vi "Autonomous Independent.vi"() -> ()   [LabVIEW 2017]
doc: "This VI is called when autonomous begins, and will automatically be terminated when autonomous ends. You can carry out timed or sensor driven robot movement independently without needing to return to the caller."
uses:
  <vilib>/Rock Robotics/WPI/Solenoid/WPI_SolenoidValue.ctl
  <vilib>/Rock Robotics/WPI/Utilities/WPI_GetSetVariantRefNum.vi
  <vilib>/Rock Robotics/Network Tables/NT Read String.vi
  <vilib>/Rock Robotics/Network Tables/NT Write Numeric Array.vi
  <vilib>/Rock Robotics/WPI/Solenoid/WPI_SolenoidSetEnum.vi
  Desktop/2018 FINAL/E/2018 FINAL/C/Users/admin/Documents/LabVIEW Data/2018 FINAL CODE/Robot Global Data.vi
  <vilib>/addons/control/pid/pid.llb/PID (DBL).vi
  <vilib>/Rock Robotics/WPI/RobotDrive/WPI_RobotDriveArcadeDrive_Standard(NoSaturation).vi
  <vilib>/addons/control/pid/NI_PID_pid.lvlib
panel:
  out "Place 2 Scale":bool
  out "Place 1 Scale":bool
  out "Robots Decision 2":string
  out "Place Switch and Scale":bool
  out "Place 2 Switch":bool
  out "Center Place 1 Switch":bool
  out "Game Data":string
  out "Right":bool
  out "Center":bool
  out "Left":bool
  # "Be sure to right-click and choose Data Operations>>Make Current Value default if you want to save the array values with the VI"
types:
  T1 = enum16{"Drive Forward", "None", "Right", "Center", "Left"}
  T2 = typedef "WPI_JoystickDevRef.ctl" = cluster{"Device":T3}
  T3 = typedef "WPI_JoystickDeviceEnum.ctl" = enum16{"USB 0", "USB 1", "USB 2", "USB 3", "USB 4", "USB 5"}
  T4 = enum16{"Place 2 Scale Left", "Place 2 Scale Right", "Place Scale Right", "Place Switch and Scale Right", "Place 2 Switch Right", "Center Place 2 Switch Right", "Center Place 1 Switch Right", "Center Place 2 Switch Left", "Center Place 1 Switch Left", "Place Scale Left", "Place Switch and Scale Left", "Place 2 Switch Left", "Drive forward", "Do Nothing"}
  T5 = enum16{"Place 2 Scale", "Place 1 Scale", "Place Switch and Scale", "Place 2 Switch", "Center Place 2 Switch", "Center Place 1 Switch", "None"}
  T6 = typedef "WPI_SolenoidValue.ctl" = enum16{"Off", "On", "Forward", "Reverse"}
  T7 = cluster{"proportional gain (Kc)":dbl, "integral time (Ti, min)":dbl, "derivative time (Td, min)":dbl}
  T8 = typedef "WPI_RobotDriveDevRef.ctl" = cluster{"DevStatus":errorcluster, "Motors[]":T9[], "Square Inputs":bool, "Max Output":dbl}
  T9 = typedef "WPI_MotorControlDeviceRef.ctl" = cluster{"DeviceStatus":errorcluster, "Type":T10, "PWM":cluster{"PWM Channel":T11, "DeadBand":T12}, "CAN":cluster{"Device Number":u8, "SetOutput VI Ref":variant, "GetOutput VI Ref":variant, "Enable VI Ref":variant, "Disable VI Ref":variant, "Data":variant}, "Invert":bool, "DIO PWM":cluster{"PWM \"Enable\" Channel":T11, "DIOChannel":T13, "PWM Rate":dbl}}
  T10 = typedef "WPI_MotorControlType.ctl" = enum16{"PWM", "CAN", "DIO PWM"}
  T11 = typedef "FPGA_DIOPWMChannel.ctl" = enum8{"PWM 0", "PWM 1", "PWM 2", "PWM 3", "PWM 4", "PWM 5", "PWM 6", "PWM 7", "PWM 8", "PWM 9", "PWM MXP 0", "PWM MXP 1", "PWM MXP 2", "PWM MXP 3", "PWM MXP 4", "PWM MXP 5", "PWM MXP 6", "PWM MXP 7", "PWM MXP 8", "PWM MXP 9", "Invalid"}
  T12 = typedef "WPI_PWMDeadband.ctl" = cluster{"Name":string, "maxPositivePwm":i32, "minPositivePwm":i32, "centerPwm":i32, "maxNegativePwm":i32, "minNegativePwm":i32, "angularRange":u16}
  T13 = typedef "FPGA_DIOChannel.ctl" = enum8{"DIO 0", "DIO 1", "DIO 2", "DIO 3", "DIO 4", "DIO 5", "DIO 6", "DIO 7", "DIO 8", "DIO 9", "DIO MXP 0", "DIO MXP 1", "DIO MXP 2", "DIO MXP 3", "DIO MXP 4", "DIO MXP 5", "DIO MXP 6", "DIO MXP 7", "DIO MXP 8", "DIO MXP 9", "DIO MXP 10", "DIO MXP 11", "DIO MXP 12", "DIO MXP 13", "DIO MXP 14", "DIO MXP 15", "SPI Port CS1", "SPI Port CS2", "SPI Port CS3", "SPI Port MISO", "SPI Port MOSI", "Invalid"}
  T14 = typedef "CTRE_PigeonIMU_DeviceRef.ctl" = cluster{"DeviceStatus":errorcluster, "Device Number":u8, "Type":T15, "Device ID":u32, "Handle":u64, "UsageFrame":u32, "Library Path":path}
  T15 = typedef "CTRE_PigeonIMU_ConnectionType.ctl" = u32
  T16 = typedef "WPI_SolenoidDevRef.ctl" = cluster{"DevStatus":errorcluster, "Pneumatics Control Module":u8, "Forward Solenoid Channel":T17, "Reverse Solenoid Channel":T17}
  T17 = typedef "WPI_SolenoidChannel.ctl" = enum8{"Solenoid 0", "Solenoid 1", "Solenoid 2", "Solenoid 3", "Solenoid 4", "Solenoid 5", "Solenoid 6", "Solenoid 7", "Invalid"}
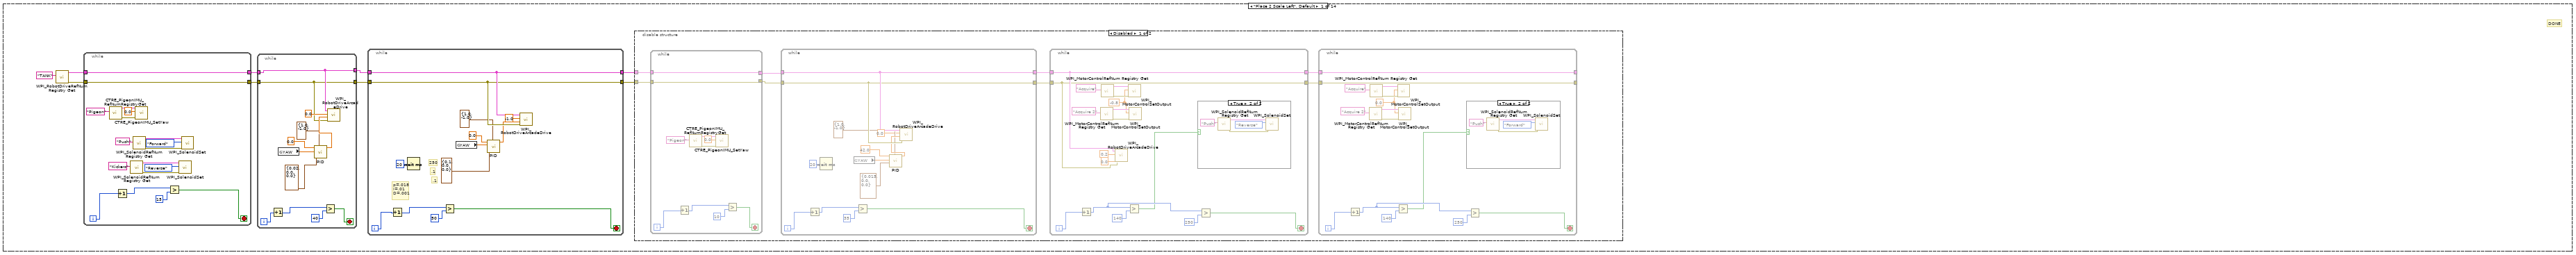
[diagram p2: hidden frame]
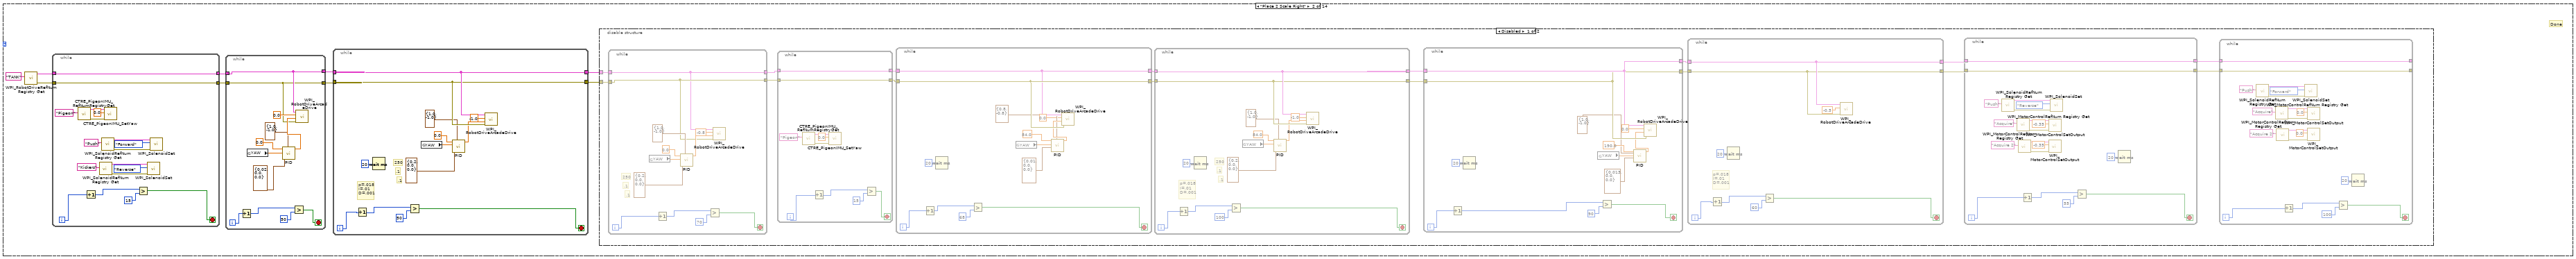
[diagram p6: hidden frame]
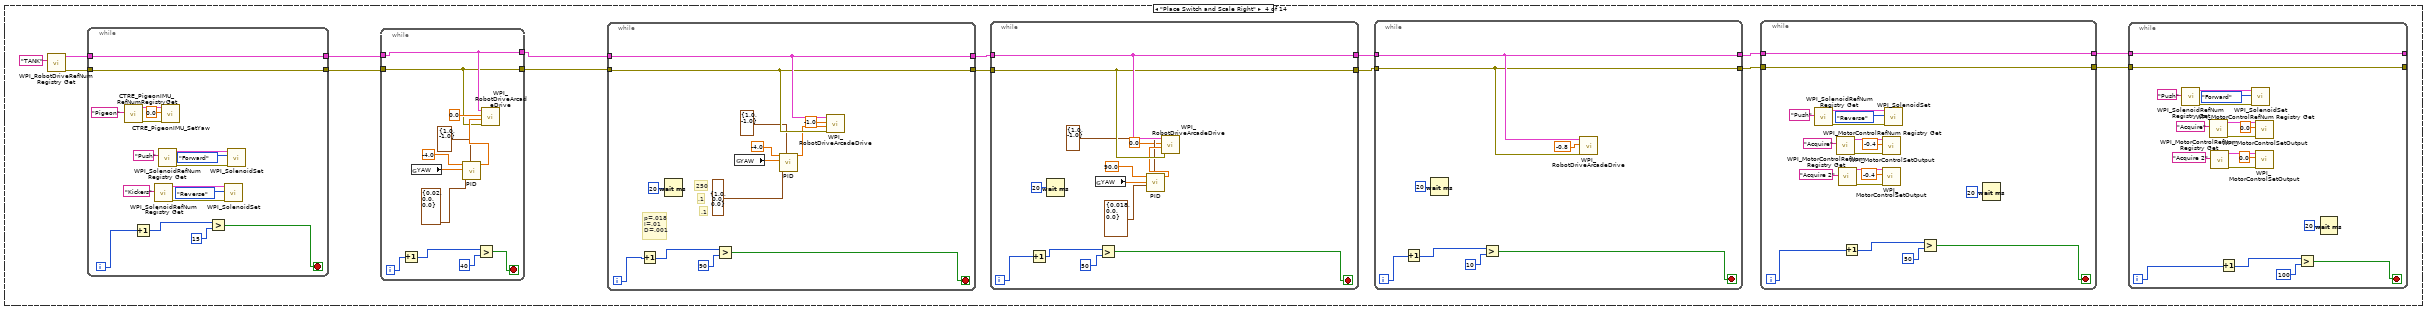
[diagram p10: hidden frame]
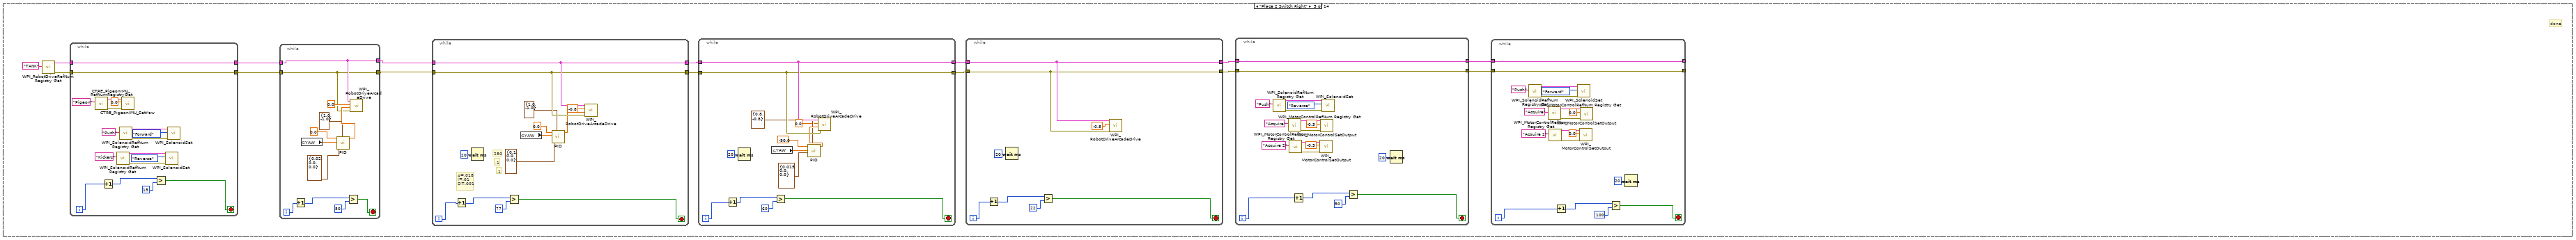
[diagram p11: hidden frame]
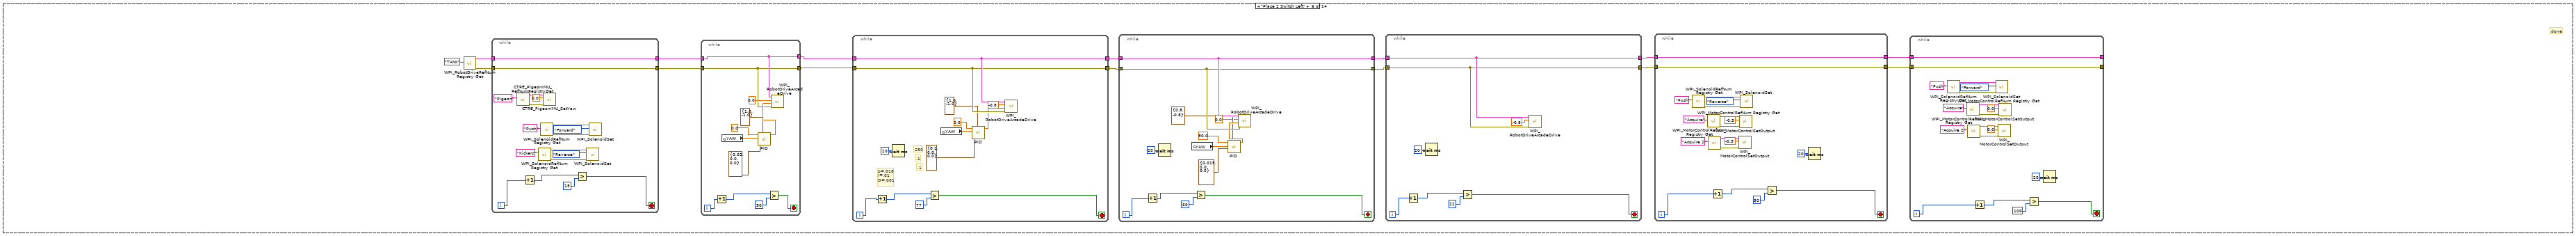
[diagram p12: hidden frame]
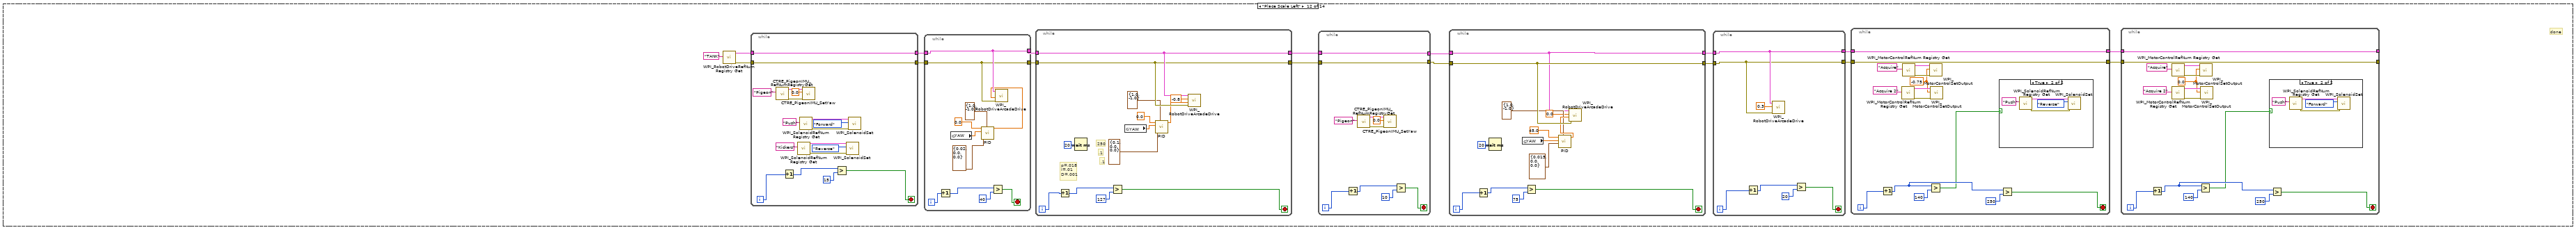
[diagram p18: hidden frame]
diagram:
  (unwired) "This function is run in parallel when the autonomous period begins. It will be terminated automatically when the period ends.\n\nNote that all Driver Station inputs are automatically latched and will not change once auto begins."
  # "5"
  # "LOGIC ALGORITHM"
  # "ALL AUTON STEPS GOES HERE"
  # "Players Choice"
  # "Order of difficulty"
  # "4"
  # "3"
  # "2"
  # "1"
  # "Game Data"
  # "Position"
  # "Position"
  # "LOGIC ALGORITHM"
  # "ALL AUTON STEPS GOES HERE"
  # "Position"
  # "This tells you the autonomous selected\nfrom the dashboard"
  # "Every 20ms, report that we are running autonomous\ncode. Loop will abort the same time as the VI."
  # "This gives you the joystick value\nthat is often the throttle"
  # "This tells you the driver position\nand alliance color"
  # "Possibilities"
  n1 = call <vilib>:"WPI_JoystickRefNum Registry Get.vi"("refnum name"="Auton") -> ("error out"=w43:errorcluster, "JoystickDevRef"=w44:T2)  [unwired: 9 in]
  n2 = call <vilib>:"WPI_JoystickGetValues.vi"("error in (no error)"=w43, "JoystickDevRef"=w44) -> ("Buttons"=w41:bool[])  [unwired: 5 in, 4 out]
  n3 = Index Array(array=w41) -> (element #1=w9:bool, element #2=w8:bool, element #4=w6:bool, element #5=w7:bool, element #10=w2:bool, element #11=w3:bool, element #13=w1:bool, element #14=w5:bool, element #16=w4:bool)  [unwired: 19 in, 10 out]
  "Left" <- w9
  "Center" <- w8
  "Right" <- w7
  "Center Place 1 Switch" <- w3
  "Place 2 Switch" <- w6
  "Place Switch and Scale" <- w2
  "Place 1 Scale" <- w5
  "Place 2 Scale" <- w4
  n4 = call <vilib>:"WPI_DriverStationGame Specific Data.vi"() -> ("Game Specific Data"=w10:string)  [unwired: 11 in]
  "Game Data" <- w10
  n5 = Select(t=T1."Right", s=w7, f=T1."None") -> (s? t:f=w37:T1)
  n6 = String Subset(string=w10, length (rest)=2 ("length (rest)")) -> (substring=w32:string)  [unwired: 1 in]
  n7 = Select(t=T1."Center", s=w8, f=w37) -> (s? t:f=w38:T1)
  n8 = Equal?(x=w32, y="RL") -> (x = y?=w26:bool)
  n9 = Equal?(x=w32, y="LR") -> (x = y?=w25:bool)
  n10 = Equal?(x=w32, y="LL") -> (x = y?=w28:bool)
  n11 = Equal?(x=w32, y="RR") -> (x = y?=w27:bool)
  n12 = Select(t=T1."Left", s=w9, f=w38) -> (s? t:f=w15:T1)
  n13 = Select(t=enum16{"None", "LR", "RL", "LL", "RR"}."LR", s=w25, f=enum16{"None", "LR", "RL", "LL", "RR"}."None") -> (s? t:f=w22:enum16{"None", "LR", "RL", "LL", "RR"})
  n14 = Select(t=enum16{"None", "LR", "RL", "LL", "RR"}."RL", s=w26, f=w22) -> (s? t:f=w23:enum16{"None", "LR", "RL", "LL", "RR"})
  n15 = Select(t=enum16{"None", "LR", "RL", "LL", "RR"}."RR", s=w27, f=w23) -> (s? t:f=w24:enum16{"None", "LR", "RL", "LL", "RR"})
  n16 = Select(t=enum16{"None", "LR", "RL", "LL", "RR"}."LL", s=w28, f=w24) -> (s? t:f=w16:enum16{"None", "LR", "RL", "LL", "RR"})
  n17 = Select(t=T1."Drive Forward", s=w1, f=w15) -> (s? t:f=w13:T1)
  n18 = case shown="\"Left\"" w13 {
    tunnel: w16 -> [_ _ w59 w163 w267]
    tunnel: w3 -> [_ _ w56 w159 w266]
    tunnel: w6 -> [_ _ w57 w160 w265]
    tunnel: w5 -> [_ _ w55 w161 w264]
    tunnel: w2 -> [_ _ w58 w162 w263]
    tunnel: w4 -> [_ _ w54 w157 w261]
    tunnel: [T4."Drive forward" T4."Do Nothing" w53 w158 w262] -> w11
    frame "Drive Forward", Default {
      # "Drive Forward code goes here. This is because drive forward can be done in any position on the field"
    }
    frame "None" {
      # "Nothing goes here."
    }
    frame "Right" {
      # "Game Data"
      n19 = case shown="\"LR\"" w59 {
        tunnel: w58 -> [w68 w88 w114 w134 _]
        tunnel: w55 -> [w73 w86 w112 w136 _]
        tunnel: w57 -> [w72 w85 w111 w137 _]
        tunnel: w56 -> [w71 w84 w110 w138 _]
        tunnel: w54 -> [w67 w87 w113 w135 _]
        tunnel: [w61 w89 w109 w132 T4."Do Nothing"] -> w53
        frame "RR" {
          # "Can do any auton"
          # "Right RR"
          n20 = Select(t=T5."Place Switch and Scale", s=w68, f=T5."None") -> (s? t:f=w69:T5)
          n21 = Select(t=T5."Place 2 Scale", s=w67, f=w69) -> (s? t:f=w76:T5)
          n22 = Select(t=T5."Place 1 Scale", s=w73, f=w76) -> (s? t:f=w75:T5)
          n23 = Select(t=T5."Place 2 Switch", s=w72, f=w75) -> (s? t:f=w74:T5)
          n24 = Select(t=T5."Place 1 Scale", s=w71, f=w74) -> (s? t:f=w70:T5)
          n25 = case shown="\"Place 2 Switch\"" w70 {
            tunnel: [T4."Place 2 Scale Right" T4."Place Scale Right" T4."Place Switch and Scale Right" T4."Place 2 Switch Right" T4."Do Nothing" T4."Do Nothing" T4."Do Nothing"] -> w61
            frame "Place 2 Scale", Default {
            }
            frame "Place 1 Scale" {
              # "Right switch"
            }
            frame "Place Switch and Scale" {
              # "Right Switch"
            }
            frame "Place 2 Switch" {
              # "Right Scale"
            }
            frame "Center Place 2 Switch" {
              # "Right Side"
            }
            frame "Center Place 1 Switch" {
            }
            frame "None" {
            }
          }
        }
        frame "LL" {
          # "Can do any auton"
          # "You can not score a cube so drive forward code goes here"
          # "Right LL"
          n26 = Select(t=T5."Place 2 Scale", s=w88, f=T5."None") -> (s? t:f=w96:T5)
          n27 = Select(t=T5."Place 2 Scale", s=w87, f=w96) -> (s? t:f=w100:T5)
          n28 = Select(t=T5."Place 2 Scale", s=w86, f=w100) -> (s? t:f=w99:T5)
          n29 = Select(t=T5."Place 2 Scale", s=w85, f=w99) -> (s? t:f=w98:T5)
          n30 = Select(t=T5."Place 2 Scale", s=w84, f=w98) -> (s? t:f=w97:T5)
          n31 = case shown="\"Place 2 Scale\", Default" w97 {
            tunnel: [T4."Drive forward" T4."Place Scale Left" T4."Place Switch and Scale Left" T4."Place 2 Switch Left" T4."Center Place 2 Switch Right" T4."Center Place 1 Switch Right" T4."Do Nothing"] -> w89
            frame "Place 2 Scale", Default {
            }
            frame "Place 1 Scale" {
              # "Right switch"
            }
            frame "Place Switch and Scale" {
            }
            frame "Place 2 Switch" {
            }
            frame "Center Place 2 Switch" {
            }
            frame "Center Place 1 Switch" {
            }
            frame "None" {
            }
          }
        }
        frame "RL" {
          # "Can do any auton"
          # "Right RL"
          n32 = Select(t=T5."Place 2 Switch", s=w114, f=T5."None") -> (s? t:f=w120:T5)
          n33 = Select(t=T5."Place 2 Switch", s=w113, f=w120) -> (s? t:f=w124:T5)
          n34 = Select(t=T5."Place 2 Switch", s=w112, f=w124) -> (s? t:f=w123:T5)
          n35 = Select(t=T5."Place 2 Switch", s=w111, f=w123) -> (s? t:f=w122:T5)
          n36 = Select(t=T5."Place 2 Switch", s=w110, f=w122) -> (s? t:f=w121:T5)
          n37 = case shown="\"Place 2 Switch\"" w121 {
            tunnel: [T4."Place 2 Scale Right" T4."Place Scale Right" T4."Place Switch and Scale Right" T4."Place 2 Switch Right" T4."Do Nothing" T4."Do Nothing" T4."Do Nothing"] -> w109
            frame "Place 2 Scale", Default {
            }
            frame "Place 1 Scale" {
              # "Right switch"
            }
            frame "Place Switch and Scale" {
              # "Right Switch"
            }
            frame "Place 2 Switch" {
              # "Right Scale"
            }
            frame "Center Place 2 Switch" {
              # "Right Side"
            }
            frame "Center Place 1 Switch" {
            }
            frame "None" {
            }
          }
        }
        frame "LR" {
          # "Can do any auton"
          # "Right LR"
          n38 = Select(t=T5."Place 1 Scale", s=w134, f=T5."None") -> (s? t:f=w144:T5)
          n39 = Select(t=T5."Place 1 Scale", s=w135, f=w144) -> (s? t:f=w148:T5)
          n40 = Select(t=T5."Place 1 Scale", s=w136, f=w148) -> (s? t:f=w147:T5)
          n41 = Select(t=T5."Place 1 Scale", s=w137, f=w147) -> (s? t:f=w146:T5)
          n42 = Select(t=T5."Place 1 Scale", s=w138, f=w146) -> (s? t:f=w145:T5)
          n43 = case shown="\"Place 1 Scale\"" w145 {
            tunnel: [T4."Place 2 Scale Right" T4."Place Scale Right" T4."Place Switch and Scale Right" T4."Place 2 Switch Right" T4."Do Nothing" T4."Do Nothing" T4."Do Nothing"] -> w132
            frame "Place 2 Scale", Default {
            }
            frame "Place 1 Scale" {
              # "Right switch"
            }
            frame "Place Switch and Scale" {
              # "Right Switch"
            }
            frame "Place 2 Switch" {
              # "Right Scale"
            }
            frame "Center Place 2 Switch" {
              # "Right Side"
            }
            frame "Center Place 1 Switch" {
            }
            frame "None" {
            }
          }
        }
        frame "None" {
          # "Nothing goes here."
        }
      }
    }
    frame "Center" {
      # "Game Data"
      n44 = case shown="\"LR\"" w163 {
        tunnel: w162 -> [w169 w193 w214 w239 _]
        tunnel: w161 -> [w167 w191 w215 w240 _]
        tunnel: w160 -> [w166 w190 w216 w241 _]
        tunnel: w159 -> [w165 w189 w217 w242 _]
        tunnel: [w164 w188 w212 w237 T4."Do Nothing"] -> w158
        tunnel: w157 -> [w168 w192 w213 w236 _]
        frame "RR" {
          # "Can do any auton"
          # "Center RR"
          n45 = Select(t=T5."Place 2 Switch", s=w169, f=T5."None") -> (s? t:f=w176:T5)
          n46 = Select(t=T5."Place 2 Switch", s=w168, f=w176) -> (s? t:f=w180:T5)
          n47 = Select(t=T5."Place 2 Switch", s=w167, f=w180) -> (s? t:f=w179:T5)
          n48 = Select(t=T5."Place 2 Switch", s=w166, f=w179) -> (s? t:f=w178:T5)
          n49 = Select(t=T5."Center Place 1 Switch", s=w165, f=w178) -> (s? t:f=w177:T5)
          n50 = case shown="\"Place 2 Scale\", Default" w177 {
            tunnel: [T4."Place 2 Scale Right" T4."Place Scale Right" T4."Place Switch and Scale Right" T4."Center Place 2 Switch Right" T4."Center Place 2 Switch Right" T4."Center Place 1 Switch Right" T4."Do Nothing"] -> w164
            frame "Place 2 Scale", Default {
            }
            frame "Place 1 Scale" {
              # "Right switch"
            }
            frame "Place Switch and Scale" {
              # "Right Switch"
            }
            frame "Place 2 Switch" {
            }
            frame "Center Place 2 Switch" {
            }
            frame "Center Place 1 Switch" {
            }
            frame "None" {
            }
          }
        }
        frame "LL" {
          # "Can do any auton"
          # "Center LL"
          n51 = Select(t=T5."Place 2 Switch", s=w193, f=T5."None") -> (s? t:f=w200:T5)
          n52 = Select(t=T5."Place 2 Switch", s=w192, f=w200) -> (s? t:f=w204:T5)
          n53 = Select(t=T5."Place 2 Switch", s=w191, f=w204) -> (s? t:f=w203:T5)
          n54 = Select(t=T5."Place 2 Switch", s=w190, f=w203) -> (s? t:f=w202:T5)
          n55 = Select(t=T5."Center Place 1 Switch", s=w189, f=w202) -> (s? t:f=w201:T5)
          n56 = case shown="\"None\"" w201 {
            tunnel: [T4."Place 2 Scale Right" T4."Place Scale Right" T4."Place Switch and Scale Right" T4."Center Place 2 Switch Left" T4."Center Place 2 Switch Left" T4."Center Place 1 Switch Left" T4."Do Nothing"] -> w188
            frame "Place 2 Scale", Default {
            }
            frame "Place 1 Scale" {
              # "Right switch"
            }
            frame "Place Switch and Scale" {
              # "Right Switch"
            }
            frame "Place 2 Switch" {
            }
            frame "Center Place 2 Switch" {
            }
            frame "Center Place 1 Switch" {
            }
            frame "None" {
            }
          }
        }
        frame "RL" {
          # "Can do any auton"
          # "Center RL"
          n57 = Select(t=T5."Place 2 Switch", s=w214, f=T5."None") -> (s? t:f=w224:T5)
          n58 = Select(t=T5."Place 2 Switch", s=w213, f=w224) -> (s? t:f=w228:T5)
          n59 = Select(t=T5."Place 2 Switch", s=w215, f=w228) -> (s? t:f=w227:T5)
          n60 = Select(t=T5."Place 2 Switch", s=w216, f=w227) -> (s? t:f=w226:T5)
          n61 = Select(t=T5."Center Place 1 Switch", s=w217, f=w226) -> (s? t:f=w225:T5)
          n62 = case shown="\"Center Place 1 Switch\"" w225 {
            tunnel: [T4."Place 2 Scale Right" T4."Place Scale Right" T4."Place Switch and Scale Right" T4."Center Place 2 Switch Right" T4."Center Place 2 Switch Right" T4."Center Place 1 Switch Right" T4."Do Nothing"] -> w212
            frame "Place 2 Scale", Default {
            }
            frame "Place 1 Scale" {
              # "Right switch"
            }
            frame "Place Switch and Scale" {
              # "Right Switch"
            }
            frame "Place 2 Switch" {
            }
            frame "Center Place 2 Switch" {
            }
            frame "Center Place 1 Switch" {
            }
            frame "None" {
            }
          }
        }
        frame "LR" {
          # "Can do any auton"
          # "Center LR"
          n63 = Select(t=T5."Place 2 Switch", s=w239, f=T5."None") -> (s? t:f=w248:T5)
          n64 = Select(t=T5."Place 2 Switch", s=w236, f=w248) -> (s? t:f=w252:T5)
          n65 = Select(t=T5."Place 2 Switch", s=w240, f=w252) -> (s? t:f=w251:T5)
          n66 = Select(t=T5."Place 2 Switch", s=w241, f=w251) -> (s? t:f=w250:T5)
          n67 = Select(t=T5."Center Place 1 Switch", s=w242, f=w250) -> (s? t:f=w249:T5)
          n68 = case shown="\"Center Place 1 Switch\"" w249 {
            tunnel: [T4."Place 2 Scale Right" T4."Place Scale Right" T4."Place Switch and Scale Right" T4."Center Place 2 Switch Left" T4."Center Place 2 Switch Left" T4."Center Place 1 Switch Left" T4."Do Nothing"] -> w237
            frame "Place 2 Scale", Default {
            }
            frame "Place 1 Scale" {
              # "Right switch"
            }
            frame "Place Switch and Scale" {
              # "Right Switch"
            }
            frame "Place 2 Switch" {
            }
            frame "Center Place 2 Switch" {
            }
            frame "Center Place 1 Switch" {
            }
            frame "None" {
            }
          }
        }
        frame "None" {
          # "Nothing goes here."
        }
      }
    }
    frame "Left" {
      n69 = case shown="\"LR\"" w267 {
        tunnel: w266 -> [w269 w292 w316 w340 _]
        tunnel: w265 -> [w270 w293 w317 w341 _]
        tunnel: w264 -> [w271 w294 w318 w342 _]
        tunnel: w263 -> [w273 w296 w320 w344 _]
        tunnel: [w268 w297 w321 w345 T4."Do Nothing"] -> w262
        tunnel: w261 -> [w272 w295 w319 w343 _]
        frame "RR" {
          # "Can do any auton"
          # "place 2 scale= drive across switch"
          # "Game Data"
          # "You can not score a cube so drive forward code goes here"
          # "Left RR"
          n70 = Select(t=T5."Place 2 Scale", s=w273, f=T5."None") -> (s? t:f=w280:T5)
          n71 = Select(t=T5."Place 2 Scale", s=w272, f=w280) -> (s? t:f=w284:T5)
          n72 = Select(t=T5."Place 2 Scale", s=w271, f=w284) -> (s? t:f=w283:T5)
          n73 = Select(t=T5."Place 2 Scale", s=w270, f=w283) -> (s? t:f=w282:T5)
          n74 = Select(t=T5."Place 2 Scale", s=w269, f=w282) -> (s? t:f=w281:T5)
          n75 = case shown="\"Place 2 Scale\", Default" w281 {
            tunnel: [T4."Drive forward" T4."Place Scale Left" T4."Place Switch and Scale Left" T4."Place 2 Switch Left" T4."Center Place 2 Switch Right" T4."Center Place 1 Switch Right" T4."Place 2 Scale Right"] -> w268
            frame "Place 2 Scale", Default {
            }
            frame "Place 1 Scale" {
              # "Right switch"
            }
            frame "Place Switch and Scale" {
            }
            frame "Place 2 Switch" {
            }
            frame "Center Place 2 Switch" {
            }
            frame "Center Place 1 Switch" {
            }
            frame "None" {
            }
          }
        }
        frame "LL" {
          # "Can do any auton"
          # "Left LL"
          n76 = Select(t=T5."Place Switch and Scale", s=w296, f=T5."None") -> (s? t:f=w304:T5)
          n77 = Select(t=T5."Place 2 Scale", s=w295, f=w304) -> (s? t:f=w308:T5)
          n78 = Select(t=T5."Place 1 Scale", s=w294, f=w308) -> (s? t:f=w307:T5)
          n79 = Select(t=T5."Place 2 Switch", s=w293, f=w307) -> (s? t:f=w306:T5)
          n80 = Select(t=T5."Place Switch and Scale", s=w292, f=w306) -> (s? t:f=w305:T5)
          n81 = case shown="\"Place 2 Switch\"" w305 {
            tunnel: [T4."Place 2 Scale Left" T4."Place Scale Left" T4."Place Switch and Scale Left" T4."Place 2 Switch Left" T4."Center Place 2 Switch Right" T4."Center Place 1 Switch Right" T4."Do Nothing"] -> w297
            frame "Place 2 Scale", Default {
            }
            frame "Place 1 Scale" {
              # "Right switch"
            }
            frame "Place Switch and Scale" {
            }
            frame "Place 2 Switch" {
            }
            frame "Center Place 2 Switch" {
            }
            frame "Center Place 1 Switch" {
            }
            frame "None" {
            }
          }
        }
        frame "RL" {
          # "Can do any auton"
          # "Left RL"
          n82 = Select(t=T5."Place 1 Scale", s=w320, f=T5."None") -> (s? t:f=w328:T5)
          n83 = Select(t=T5."Place 1 Scale", s=w319, f=w328) -> (s? t:f=w332:T5)
          n84 = Select(t=T5."Place 1 Scale", s=w318, f=w332) -> (s? t:f=w331:T5)
          n85 = Select(t=T5."Place 1 Scale", s=w317, f=w331) -> (s? t:f=w330:T5)
          n86 = Select(t=T5."Place 1 Scale", s=w316, f=w330) -> (s? t:f=w329:T5)
          n87 = case shown="\"Place 1 Scale\"" w329 {
            tunnel: [T4."Place 2 Scale Left" T4."Place Scale Left" T4."Place Switch and Scale Right" T4."Place 2 Switch Left" T4."Center Place 2 Switch Right" T4."Center Place 1 Switch Right" T4."Do Nothing"] -> w321
            frame "Place 2 Scale", Default {
            }
            frame "Place 1 Scale" {
              # "Right switch"
            }
            frame "Place Switch and Scale" {
              # "Right Switch"
            }
            frame "Place 2 Switch" {
            }
            frame "Center Place 2 Switch" {
            }
            frame "Center Place 1 Switch" {
            }
            frame "None" {
            }
          }
        }
        frame "LR" {
          # "Can do any auton"
          # "Left LR"
          n88 = Select(t=T5."Place 2 Switch", s=w344, f=T5."None") -> (s? t:f=w352:T5)
          n89 = Select(t=T5."Place 2 Switch", s=w343, f=w352) -> (s? t:f=w356:T5)
          n90 = Select(t=T5."Place 2 Switch", s=w342, f=w356) -> (s? t:f=w355:T5)
          n91 = Select(t=T5."Place 2 Switch", s=w341, f=w355) -> (s? t:f=w354:T5)
          n92 = Select(t=T5."Place 2 Switch", s=w340, f=w354) -> (s? t:f=w353:T5)
          n93 = case shown="\"Place 2 Switch\"" w353 {
            tunnel: [T4."Place 2 Scale Right" T4."Place Scale Right" T4."Place Switch and Scale Right" T4."Place 2 Switch Left" T4."Center Place 2 Switch Right" T4."Center Place 1 Switch Right" T4."Do Nothing"] -> w345
            frame "Place 2 Scale", Default {
            }
            frame "Place 1 Scale" {
              # "Right switch"
            }
            frame "Place Switch and Scale" {
              # "Right Switch"
            }
            frame "Place 2 Switch" {
            }
            frame "Center Place 2 Switch" {
            }
            frame "Center Place 1 Switch" {
            }
            frame "None" {
            }
          }
        }
        frame "None" {
          # "Nothing goes here."
        }
      }
    }
  }
  n94 = case shown="\"Place Scale Right\"" w11 {
    frame "Place 2 Scale Left", Default {
      # "DONE"
      n95 = call <vilib>:"WPI_RobotDriveRefNum Registry Get.vi"("refnum name"="TANK") -> ("error out"=w371:errorcluster, "RobotDriveDevRef"=w372:T8)  [unwired: 9 in]
      n96 = while {
        tunnel: [w474] -> w368
        tunnel: w372 -> [w474]
        tunnel: w371 -> [w473]
        tunnel: [w473] -> w366
        i -> [w470]
        stop <- w469 stop-if-true
        n97 = call <vilib>:"CTRE_PigeonIMU_RefNumRegistryGet.vi"("refnum name"="Pigeon") -> ("error out"=w466:errorcluster, "PigeonIMUDevRef"=w467:T14)  [unwired: 9 in]
        n98 = Increment(x=w470) -> (x+1=w471:i32)
        n99 = call <vilib>:"WPI_SolenoidRefNum Registry Get.vi"("refnum name"="Kickers") -> ("error out"=w458:errorcluster, "SolenoidDevRef"=w459:T16)  [unwired: 9 in]
        n100 = call <vilib>:"WPI_SolenoidRefNum Registry Get.vi"("refnum name"="Push") -> ("error out"=w462:errorcluster, "SolenoidDevRef"=w463:T16)  [unwired: 9 in]
        n101 = call <vilib>:"CTRE_PigeonIMU_SetYaw.vi"("error in (no error)"=w466, "Value"=0.0, "PigeonIMUDevRef"=w467) -> ()  [unwired: 7 in, 2 out]
        n102 = Greater?(x=w471, y=15) -> (0:w469:bool)
        n103 = call-poly <vilib>:"WPI_SolenoidSet.vi"("error in (no error)"=w458, "Value"=WPI_SolenoidValue."Reverse", "SolenoidDevRef"=w459) -> ()  [unwired: 7 in, 2 out]
        n104 = call-poly <vilib>:"WPI_SolenoidSet.vi"("error in (no error)"=w462, "Value"=WPI_SolenoidValue."Forward", "SolenoidDevRef"=w463) -> ()  [unwired: 7 in, 2 out]
      }
      n105 = while {
        tunnel: w368 -> [w446]
        tunnel: [w446] -> w367
        tunnel: w366 -> [w445]
        tunnel: [w445] -> w365
        i -> [w448]
        stop <- w447 stop-if-true
        n106 = Increment(x=w448) -> (x+1=w449:i32)
        n107 = global read "Robot Global Data.vi" "YAW"() -> (w454:dbl)
        n108 = call-poly <vilib>:"PID.vi"("output range"=cluster{"output high":dbl, "output low":dbl} {"output high"=1.0, "output low"=-1.0}, "PID gains"=T7 {"proportional gain (Kc)"=0.02, "integral time (Ti, min)"=0.0, "derivative time (Td, min)"=0.0}, "process variable"=w454, "setpoint"=0.0) -> ("output"=w453:dbl)  [unwired: 6 in, 1 out]
        n109 = Greater?(x=w449, y=40) -> (0:w447:bool)
        n110 = call-poly <vilib>:"WPI_RobotDriveArcadeDrive.vi"("error in (no error)"=w445, "Y axis value"=w453, "X axis value"=0.0, "RobotDriveDevRef"=w446) -> ()  [unwired: 5 in, 3 out]
      }
      n111 = while {
        tunnel: w367 -> [w482]
        tunnel: w365 -> [w481]
        tunnel: [w482] -> w370
        tunnel: [w481] -> w369
        i -> [w484]
        stop <- w487 stop-if-true
        # ".1"
        # ".1"
        # "250"
        # "p=.018\nI=.01\nD=.001"
        n112 = Increment(x=w484) -> (x+1=w483:i32)
        n113 = Wait (ms)(milliseconds to wait=u32 20) -> ()  [unwired: 1 out]
        n114 = Greater?(x=w483, y=50) -> (0:w487:bool)
        n115 = global read "Robot Global Data.vi" "YAW"() -> (w478:dbl)
        n116 = call-poly <vilib>:"PID.vi"("output range"=cluster{"output high":dbl, "output low":dbl} {"output high"=1.0, "output low"=-1.0}, "PID gains"=T7 {"proportional gain (Kc)"=0.1, "integral time (Ti, min)"=0.0, "derivative time (Td, min)"=0.0}, "process variable"=w478, "setpoint"=0.0) -> ("output"=w476:dbl)  [unwired: 6 in, 1 out]
        n117 = call-poly <vilib>:"WPI_RobotDriveArcadeDrive.vi"("error in (no error)"=w481, "Y axis value"=w476, "X axis value"=-1.0, "RobotDriveDevRef"=w482) -> ()  [unwired: 5 in, 3 out]
      }
      n118 = disable-structure shown="Disabled" {
        disable-tunnel: w370 -> [w379 _]
        disable-tunnel: w369 -> [w378 _]
        frame Disabled {
          n119 = while {
            tunnel: w379 -> [w409]
            tunnel: w378 -> [w410]
            tunnel: [w410] -> w377
            tunnel: [w409] -> w376
            i -> [w402]
            stop <- w401 stop-if-true
            n120 = Increment(x=w402) -> (x+1=w404:i32)
            n121 = call <vilib>:"CTRE_PigeonIMU_RefNumRegistryGet.vi"("refnum name"="Pigeon") -> ("error out"=w406:errorcluster, "PigeonIMUDevRef"=w407:T14)  [unwired: 9 in]
            n122 = call <vilib>:"CTRE_PigeonIMU_SetYaw.vi"("error in (no error)"=w406, "Value"=0.0, "PigeonIMUDevRef"=w407) -> ()  [unwired: 7 in, 2 out]
            n123 = Greater?(x=w404, y=10) -> (0:w401:bool)
          }
          n124 = while {
            tunnel: w376 -> [w439]
            tunnel: w377 -> [w438]
            tunnel: [w439] -> w381
            tunnel: [w438] -> w380
            i -> [w444]
            stop <- w443 stop-if-true
            n125 = Increment(x=w444) -> (x+1=w441:i32)
            n126 = Wait (ms)(milliseconds to wait=u32 20) -> ()  [unwired: 1 out]
            n127 = global read "Robot Global Data.vi" "YAW"() -> (w435:dbl)
            n128 = Greater?(x=w441, y=35) -> (0:w443:bool)
            n129 = call-poly <vilib>:"PID.vi"("output range"=cluster{"output high":dbl, "output low":dbl} {"output high"=1.0, "output low"=-1.0}, "PID gains"=T7 {"proportional gain (Kc)"=0.015, "integral time (Ti, min)"=0.0, "derivative time (Td, min)"=0.0}, "process variable"=w435, "setpoint"=42.0) -> ("output"=w434:dbl)  [unwired: 6 in, 1 out]
            n130 = call-poly <vilib>:"WPI_RobotDriveArcadeDrive.vi"("error in (no error)"=w438, "Y axis value"=w434, "X axis value"=0.0, "RobotDriveDevRef"=w439) -> ()  [unwired: 5 in, 3 out]
          }
          n131 = while {
            tunnel: w381 -> [w412]
            tunnel: w380 -> [w411]
            tunnel: [w412] -> w375
            tunnel: [w411] -> w374
            i -> [w427]
            stop <- w416 stop-if-true
            w419 = -0.8
            n132 = Increment(x=w427) -> (x+1=w417:i32)
            n133 = call <vilib>:"WPI_MotorControlRefNum Registry Get.vi"("refnum name"="Acquire 2") -> ("error out"=w420:errorcluster, "MotorControlDevRef"=w421:T9)  [unwired: 9 in]
            n134 = call <vilib>:"WPI_MotorControlRefNum Registry Get.vi"("refnum name"="Acquire") -> ("error out"=w423:errorcluster, "MotorControlDevRef"=w424:T9)  [unwired: 9 in]
            n135 = call-poly <vilib>:"WPI_RobotDriveArcadeDrive.vi"("error in (no error)"=w411, "Y axis value"=0.0, "X axis value"=0.2, "RobotDriveDevRef"=w412) -> ()  [unwired: 5 in, 3 out]
            n136 = Greater?(x=w417, y=140) -> (0:w415:bool)
            n137 = call <vilib>:"WPI_MotorControlSetOutput.vi"("error in (no error)"=w423, "Output"=w419, "MotorControlDevRef"=w424) -> ()  [unwired: 6 in, 3 out]
            n138 = call <vilib>:"WPI_MotorControlSetOutput.vi"("error in (no error)"=w420, "Output"=w419, "MotorControlDevRef"=w421) -> ()  [unwired: 6 in, 3 out]
            n139 = case shown="True" w415 {
              frame False {
              }
              frame True {
                n140 = call <vilib>:"WPI_SolenoidRefNum Registry Get.vi"("refnum name"="Push") -> ("error out"=w429:errorcluster, "SolenoidDevRef"=w430:T16)  [unwired: 9 in]
                n141 = call-poly <vilib>:"WPI_SolenoidSet.vi"("error in (no error)"=w429, "Value"=WPI_SolenoidValue."Reverse", "SolenoidDevRef"=w430) -> ()  [unwired: 7 in, 2 out]
              }
            }
            n142 = Greater?(x=w417, y=250) -> (0:w416:bool)
          }
          n143 = while {
            tunnel: w375 -> [w383]
            tunnel: w374 -> [w382]
            tunnel: [w383] -> _
            tunnel: [w382] -> _
            i -> [w396]
            stop <- w385 stop-if-true
            w388 = 0.0
            n144 = Increment(x=w396) -> (x+1=w386:i32)
            n145 = call <vilib>:"WPI_MotorControlRefNum Registry Get.vi"("refnum name"="Acquire 2") -> ("error out"=w389:errorcluster, "MotorControlDevRef"=w390:T9)  [unwired: 9 in]
            n146 = call <vilib>:"WPI_MotorControlRefNum Registry Get.vi"("refnum name"="Acquire") -> ("error out"=w392:errorcluster, "MotorControlDevRef"=w393:T9)  [unwired: 9 in]
            n147 = Greater?(x=w386, y=140) -> (0:w384:bool)
            n148 = call <vilib>:"WPI_MotorControlSetOutput.vi"("error in (no error)"=w392, "Output"=w388, "MotorControlDevRef"=w393) -> ()  [unwired: 6 in, 3 out]
            n149 = call <vilib>:"WPI_MotorControlSetOutput.vi"("error in (no error)"=w389, "Output"=w388, "MotorControlDevRef"=w390) -> ()  [unwired: 6 in, 3 out]
            n150 = case shown="True" w384 {
              frame False {
              }
              frame True {
                n151 = call <vilib>:"WPI_SolenoidRefNum Registry Get.vi"("refnum name"="Push") -> ("error out"=w398:errorcluster, "SolenoidDevRef"=w399:T16)  [unwired: 9 in]
                n152 = call-poly <vilib>:"WPI_SolenoidSet.vi"("error in (no error)"=w398, "Value"=WPI_SolenoidValue."Forward", "SolenoidDevRef"=w399) -> ()  [unwired: 7 in, 2 out]
              }
            }
            n153 = Greater?(x=w386, y=250) -> (0:w385:bool)
          }
        }
        frame Enabled {
        }
      }
    }
    frame "Place 2 Scale Right" {
      # "Done"
      n154 = call <vilib>:"WPI_RobotDriveRefNum Registry Get.vi"("refnum name"="TANK") -> ("error out"=w494:errorcluster, "RobotDriveDevRef"=w495:T8)  [unwired: 9 in]
      n155 = while {
        tunnel: [w649] -> w493
        tunnel: w495 -> [w649]
        tunnel: w494 -> [w648]
        tunnel: [w648] -> w492
        i -> [w645]
        stop <- w644 stop-if-true
        n156 = call <vilib>:"CTRE_PigeonIMU_RefNumRegistryGet.vi"("refnum name"="Pigeon") -> ("error out"=w641:errorcluster, "PigeonIMUDevRef"=w642:T14)  [unwired: 9 in]
        n157 = Increment(x=w645) -> (x+1=w646:i32)
        n158 = call <vilib>:"WPI_SolenoidRefNum Registry Get.vi"("refnum name"="Kickers") -> ("error out"=w633:errorcluster, "SolenoidDevRef"=w634:T16)  [unwired: 9 in]
        n159 = call <vilib>:"WPI_SolenoidRefNum Registry Get.vi"("refnum name"="Push") -> ("error out"=w637:errorcluster, "SolenoidDevRef"=w638:T16)  [unwired: 9 in]
        n160 = call <vilib>:"CTRE_PigeonIMU_SetYaw.vi"("error in (no error)"=w641, "Value"=0.0, "PigeonIMUDevRef"=w642) -> ()  [unwired: 7 in, 2 out]
        n161 = Greater?(x=w646, y=15) -> (0:w644:bool)
        n162 = call-poly <vilib>:"WPI_SolenoidSet.vi"("error in (no error)"=w633, "Value"=WPI_SolenoidValue."Reverse", "SolenoidDevRef"=w634) -> ()  [unwired: 7 in, 2 out]
        n163 = call-poly <vilib>:"WPI_SolenoidSet.vi"("error in (no error)"=w637, "Value"=WPI_SolenoidValue."Forward", "SolenoidDevRef"=w638) -> ()  [unwired: 7 in, 2 out]
      }
      n164 = while {
        tunnel: w493 -> [w621]
        tunnel: [w621] -> w491
        tunnel: w492 -> [w620]
        tunnel: [w620] -> w490
        i -> [w623]
        stop <- w622 stop-if-true
        n165 = Increment(x=w623) -> (x+1=w624:i32)
        n166 = global read "Robot Global Data.vi" "YAW"() -> (w629:dbl)
        n167 = call-poly <vilib>:"PID.vi"("output range"=cluster{"output high":dbl, "output low":dbl} {"output high"=1.0, "output low"=-1.0}, "PID gains"=T7 {"proportional gain (Kc)"=0.02, "integral time (Ti, min)"=0.0, "derivative time (Td, min)"=0.0}, "process variable"=w629, "setpoint"=0.0) -> ("output"=w628:dbl)  [unwired: 6 in, 1 out]
        n168 = Greater?(x=w624, y=50) -> (0:w622:bool)
        n169 = call-poly <vilib>:"WPI_RobotDriveArcadeDrive.vi"("error in (no error)"=w620, "Y axis value"=w628, "X axis value"=0.0, "RobotDriveDevRef"=w621) -> ()  [unwired: 5 in, 3 out]
      }
      n170 = while {
        tunnel: w491 -> [w657]
        tunnel: w490 -> [w656]
        tunnel: [w657] -> w489
        tunnel: [w656] -> w488
        i -> [w659]
        stop <- w662 stop-if-true
        # ".1"
        # ".1"
        # "250"
        # "p=.018\nI=.01\nD=.001"
        n171 = Increment(x=w659) -> (x+1=w658:i32)
        n172 = Wait (ms)(milliseconds to wait=u32 20) -> ()  [unwired: 1 out]
        n173 = Greater?(x=w658, y=50) -> (0:w662:bool)
        n174 = global read "Robot Global Data.vi" "YAW"() -> (w654:dbl)
        n175 = call-poly <vilib>:"PID.vi"("output range"=cluster{"output high":dbl, "output low":dbl} {"output high"=1.0, "output low"=-1.0}, "PID gains"=T7 {"proportional gain (Kc)"=0.2, "integral time (Ti, min)"=0.0, "derivative time (Td, min)"=0.0}, "process variable"=w654, "setpoint"=0.0) -> ("output"=w652:dbl)  [unwired: 6 in, 1 out]
        n176 = call-poly <vilib>:"WPI_RobotDriveArcadeDrive.vi"("error in (no error)"=w656, "Y axis value"=w652, "X axis value"=-1.0, "RobotDriveDevRef"=w657) -> ()  [unwired: 5 in, 3 out]
      }
      n177 = disable-structure shown="Disabled" {
        disable-tunnel: w489 -> [w500 _]
        disable-tunnel: w488 -> [w498 _]
        frame Disabled {
          n178 = while {
            tunnel: [w517] -> w499
            tunnel: w500 -> [w517]
            tunnel: w498 -> [w518]
            tunnel: [w518] -> w497
            i -> [w514]
            stop <- w513 stop-if-true
            # ".1"
            # ".1"
            # "250"
            n179 = global read "Robot Global Data.vi" "YAW"() -> (w523:dbl)
            n180 = Increment(x=w514) -> (x+1=w515:i32)
            n181 = call-poly <vilib>:"PID.vi"("output range"=cluster{"output high":dbl, "output low":dbl} {"output high"=1.0, "output low"=-1.0}, "PID gains"=T7 {"proportional gain (Kc)"=0.2, "integral time (Ti, min)"=0.0, "derivative time (Td, min)"=0.0}, "process variable"=w523, "setpoint"=0.0) -> ("output"=w521:dbl)  [unwired: 6 in, 1 out]
            n182 = Greater?(x=w515, y=70) -> (0:w513:bool)
            n183 = call-poly <vilib>:"WPI_RobotDriveArcadeDrive.vi"("error in (no error)"=w518, "Y axis value"=w521, "X axis value"=-0.8, "RobotDriveDevRef"=w517) -> ()  [unwired: 5 in, 3 out]
          }
          n184 = while {
            tunnel: [w534] -> w502
            tunnel: w499 -> [w534]
            tunnel: w497 -> [w533]
            tunnel: [w533] -> w501
            i -> [w530]
            stop <- w529 stop-if-true
            n185 = call <vilib>:"CTRE_PigeonIMU_RefNumRegistryGet.vi"("refnum name"="Pigeon") -> ("error out"=w526:errorcluster, "PigeonIMUDevRef"=w527:T14)  [unwired: 9 in]
            n186 = Increment(x=w530) -> (x+1=w531:i32)
            n187 = call <vilib>:"CTRE_PigeonIMU_SetYaw.vi"("error in (no error)"=w526, "Value"=0.0, "PigeonIMUDevRef"=w527) -> ()  [unwired: 7 in, 2 out]
            n188 = Greater?(x=w531, y=15) -> (0:w529:bool)
          }
          n189 = while {
            tunnel: w502 -> [w614]
            tunnel: w501 -> [w613]
            tunnel: [w614] -> w512
            tunnel: [w613] -> w511
            i -> [w619]
            stop <- w618 stop-if-true
            n190 = Increment(x=w619) -> (x+1=w616:i32)
            n191 = Wait (ms)(milliseconds to wait=u32 20) -> ()  [unwired: 1 out]
            n192 = Greater?(x=w616, y=68) -> (0:w618:bool)
            n193 = global read "Robot Global Data.vi" "YAW"() -> (w610:dbl)
            n194 = call-poly <vilib>:"PID.vi"("output range"=cluster{"output high":dbl, "output low":dbl} {"output high"=0.8, "output low"=-0.8}, "PID gains"=T7 {"proportional gain (Kc)"=0.01, "integral time (Ti, min)"=0.0, "derivative time (Td, min)"=0.0}, "process variable"=w610, "setpoint"=84.0) -> ("output"=w609:dbl)  [unwired: 6 in, 1 out]
            n195 = call-poly <vilib>:"WPI_RobotDriveArcadeDrive.vi"("error in (no error)"=w613, "Y axis value"=w609, "X axis value"=0.0, "RobotDriveDevRef"=w614) -> ()  [unwired: 5 in, 3 out]
          }
          n196 = while {
            tunnel: w512 -> [w601]
            tunnel: w511 -> [w600]
            tunnel: [w601] -> w510
            tunnel: [w600] -> w509
            i -> [w603]
            stop <- w606 stop-if-true
            # ".1"
            # ".1"
            # "250"
            # "p=.018\nI=.01\nD=.001"
            n197 = Increment(x=w603) -> (x+1=w602:i32)
            n198 = Wait (ms)(milliseconds to wait=u32 20) -> ()  [unwired: 1 out]
            n199 = Greater?(x=w602, y=100) -> (0:w606:bool)
            n200 = global read "Robot Global Data.vi" "YAW"() -> (w597:dbl)
            n201 = call-poly <vilib>:"PID.vi"("output range"=cluster{"output high":dbl, "output low":dbl} {"output high"=1.0, "output low"=-1.0}, "PID gains"=T7 {"proportional gain (Kc)"=0.2, "integral time (Ti, min)"=0.0, "derivative time (Td, min)"=0.0}, "process variable"=w597, "setpoint"=84.0) -> ("output"=w595:dbl)  [unwired: 6 in, 1 out]
            n202 = call-poly <vilib>:"WPI_RobotDriveArcadeDrive.vi"("error in (no error)"=w600, "Y axis value"=w595, "X axis value"=-1.0, "RobotDriveDevRef"=w601) -> ()  [unwired: 5 in, 3 out]
          }
          n203 = while {
            tunnel: w510 -> [w588]
            tunnel: w509 -> [w587]
            tunnel: [w588] -> w508
            tunnel: [w587] -> w507
            i -> [w593]
            stop <- w592 stop-if-true
            n204 = Increment(x=w593) -> (x+1=w590:i32)
            n205 = Wait (ms)(milliseconds to wait=u32 20) -> ()  [unwired: 1 out]
            n206 = global read "Robot Global Data.vi" "YAW"() -> (w584:dbl)
            n207 = Greater?(x=w590, y=90) -> (0:w592:bool)
            n208 = call-poly <vilib>:"PID.vi"("output range"=cluster{"output high":dbl, "output low":dbl} {"output high"=1.0, "output low"=-1.0}, "PID gains"=T7 {"proportional gain (Kc)"=0.013, "integral time (Ti, min)"=0.0, "derivative time (Td, min)"=0.0}, "process variable"=w584, "setpoint"=190.0) -> ("output"=w583:dbl)  [unwired: 6 in, 1 out]
            n209 = call-poly <vilib>:"WPI_RobotDriveArcadeDrive.vi"("error in (no error)"=w587, "Y axis value"=w583, "X axis value"=0.0, "RobotDriveDevRef"=w588) -> ()  [unwired: 5 in, 3 out]
          }
          n210 = while {
            tunnel: w508 -> [w575]
            tunnel: w507 -> [w574]
            tunnel: [w575] -> w504
            tunnel: [w574] -> w503
            i -> [w577]
            stop <- w580 stop-if-true
            # "p=.018\nI=.01\nD=.001"
            n211 = Increment(x=w577) -> (x+1=w576:i32)
            n212 = Wait (ms)(milliseconds to wait=u32 20) -> ()  [unwired: 1 out]
            n213 = Greater?(x=w576, y=60) -> (0:w580:bool)
            n214 = call-poly <vilib>:"WPI_RobotDriveArcadeDrive.vi"("error in (no error)"=w574, "X axis value"=-0.5, "RobotDriveDevRef"=w575) -> ()  [unwired: 6 in, 3 out]
          }
          n215 = while {
            tunnel: [w556] -> w506
            tunnel: w504 -> [w556]
            tunnel: [w555] -> w505
            tunnel: w503 -> [w555]
            i -> [w558]
            stop <- w557 stop-if-true
            n216 = call <vilib>:"WPI_SolenoidRefNum Registry Get.vi"("refnum name"="Push") -> ("error out"=w570:errorcluster, "SolenoidDevRef"=w571:T16)  [unwired: 9 in]
            n217 = call <vilib>:"WPI_MotorControlRefNum Registry Get.vi"("refnum name"="Acquire") -> ("error out"=w563:errorcluster, "MotorControlDevRef"=w564:T9)  [unwired: 9 in]
            n218 = call <vilib>:"WPI_MotorControlRefNum Registry Get.vi"("refnum name"="Acquire 2") -> ("error out"=w565:errorcluster, "MotorControlDevRef"=w566:T9)  [unwired: 9 in]
            n219 = Increment(x=w558) -> (x+1=w559:i32)
            n220 = call <vilib>:"WPI_MotorControlSetOutput.vi"("error in (no error)"=w565, "Output"=-0.35, "MotorControlDevRef"=w566) -> ()  [unwired: 6 in, 3 out]
            n221 = call <vilib>:"WPI_MotorControlSetOutput.vi"("error in (no error)"=w563, "Output"=-0.35, "MotorControlDevRef"=w564) -> ()  [unwired: 6 in, 3 out]
            n222 = call-poly <vilib>:"WPI_SolenoidSet.vi"("error in (no error)"=w570, "Value"=WPI_SolenoidValue."Reverse", "SolenoidDevRef"=w571) -> ()  [unwired: 7 in, 2 out]
            n223 = Greater?(x=w559, y=55) -> (0:w557:bool)
            n224 = Wait (ms)(milliseconds to wait=u32 20) -> ()  [unwired: 1 out]
          }
          n225 = while {
            tunnel: [w540] -> _
            tunnel: w506 -> [w540]
            tunnel: [w539] -> _
            tunnel: w505 -> [w539]
            i -> [w543]
            stop <- w542 stop-if-true
            n226 = call <vilib>:"WPI_SolenoidRefNum Registry Get.vi"("refnum name"="Push") -> ("error out"=w536:errorcluster, "SolenoidDevRef"=w537:T16)  [unwired: 9 in]
            n227 = call <vilib>:"WPI_MotorControlRefNum Registry Get.vi"("refnum name"="Acquire") -> ("error out"=w548:errorcluster, "MotorControlDevRef"=w549:T9)  [unwired: 9 in]
            n228 = call <vilib>:"WPI_MotorControlRefNum Registry Get.vi"("refnum name"="Acquire 2") -> ("error out"=w550:errorcluster, "MotorControlDevRef"=w551:T9)  [unwired: 9 in]
            n229 = Increment(x=w543) -> (x+1=w544:i32)
            n230 = call-poly <vilib>:"WPI_SolenoidSet.vi"("error in (no error)"=w536, "Value"=WPI_SolenoidValue."Forward", "SolenoidDevRef"=w537) -> ()  [unwired: 7 in, 2 out]
            n231 = call <vilib>:"WPI_MotorControlSetOutput.vi"("error in (no error)"=w550, "Output"=0.0, "MotorControlDevRef"=w551) -> ()  [unwired: 6 in, 3 out]
            n232 = call <vilib>:"WPI_MotorControlSetOutput.vi"("error in (no error)"=w548, "Output"=0.0, "MotorControlDevRef"=w549) -> ()  [unwired: 6 in, 3 out]
            n233 = Greater?(x=w544, y=100) -> (0:w542:bool)
            n234 = Wait (ms)(milliseconds to wait=u32 20) -> ()  [unwired: 1 out]
          }
        }
        frame Enabled {
        }
      }
    }
    frame "Place Scale Right" {
      # "done"
      n235 = call <vilib>:"WPI_RobotDriveRefNum Registry Get.vi"("refnum name"="TANK") -> ("error out"=w677:errorcluster, "RobotDriveDevRef"=w678:T8)  [unwired: 9 in]
      n236 = while {
        tunnel: [w776] -> w672
        tunnel: w678 -> [w776]
        tunnel: w677 -> [w775]
        tunnel: [w775] -> w670
        i -> [w772]
        stop <- w771 stop-if-true
        n237 = call <vilib>:"CTRE_PigeonIMU_RefNumRegistryGet.vi"("refnum name"="Pigeon") -> ("error out"=w768:errorcluster, "PigeonIMUDevRef"=w769:T14)  [unwired: 9 in]
        n238 = Increment(x=w772) -> (x+1=w773:i32)
        n239 = call <vilib>:"WPI_SolenoidRefNum Registry Get.vi"("refnum name"="Kickers") -> ("error out"=w760:errorcluster, "SolenoidDevRef"=w761:T16)  [unwired: 9 in]
        n240 = call <vilib>:"WPI_SolenoidRefNum Registry Get.vi"("refnum name"="Push") -> ("error out"=w764:errorcluster, "SolenoidDevRef"=w765:T16)  [unwired: 9 in]
        n241 = call <vilib>:"CTRE_PigeonIMU_SetYaw.vi"("error in (no error)"=w768, "Value"=0.0, "PigeonIMUDevRef"=w769) -> ()  [unwired: 7 in, 2 out]
        n242 = Greater?(x=w773, y=15) -> (0:w771:bool)
        n243 = call-poly <vilib>:"WPI_SolenoidSet.vi"("error in (no error)"=w760, "Value"=WPI_SolenoidValue."Reverse", "SolenoidDevRef"=w761) -> ()  [unwired: 7 in, 2 out]
        n244 = call-poly <vilib>:"WPI_SolenoidSet.vi"("error in (no error)"=w764, "Value"=WPI_SolenoidValue."Forward", "SolenoidDevRef"=w765) -> ()  [unwired: 7 in, 2 out]
      }
      n245 = while {
        tunnel: w672 -> [w710]
        tunnel: [w710] -> w671
        tunnel: w670 -> [w709]
        tunnel: [w709] -> w669
        i -> [w712]
        stop <- w711 stop-if-true
        n246 = Increment(x=w712) -> (x+1=w713:i32)
        n247 = global read "Robot Global Data.vi" "YAW"() -> (w707:dbl)
        n248 = call-poly <vilib>:"PID.vi"("output range"=cluster{"output high":dbl, "output low":dbl} {"output high"=1.0, "output low"=-1.0}, "PID gains"=T7 {"proportional gain (Kc)"=0.02, "integral time (Ti, min)"=0.0, "derivative time (Td, min)"=0.0}, "process variable"=w707, "setpoint"=0.0) -> ("output"=w708:dbl)  [unwired: 6 in, 1 out]
        n249 = Greater?(x=w713, y=40) -> (0:w711:bool)
        n250 = call-poly <vilib>:"WPI_RobotDriveArcadeDrive.vi"("error in (no error)"=w709, "Y axis value"=w708, "RobotDriveDevRef"=w710) -> ()  [unwired: 6 in, 3 out]
      }
      n251 = while {
        tunnel: w671 -> [w784]
        tunnel: w669 -> [w783]
        tunnel: [w784] -> w676
        tunnel: [w783] -> w675
        i -> [w786]
        stop <- w789 stop-if-true
        # ".1"
        # ".1"
        # "250"
        # "p=.018\nI=.01\nD=.001"
        n252 = Increment(x=w786) -> (x+1=w785:i32)
        n253 = Wait (ms)(milliseconds to wait=u32 20) -> ()  [unwired: 1 out]
        n254 = Greater?(x=w785, y=127) -> (0:w789:bool)
        n255 = global read "Robot Global Data.vi" "YAW"() -> (w777:dbl)
        n256 = call-poly <vilib>:"PID.vi"("output range"=cluster{"output high":dbl, "output low":dbl} {"output high"=1.0, "output low"=-1.0}, "PID gains"=T7 {"proportional gain (Kc)"=0.1, "integral time (Ti, min)"=0.0, "derivative time (Td, min)"=0.0}, "process variable"=w777, "setpoint"=0.0) -> ("output"=w779:dbl)  [unwired: 6 in, 1 out]
        n257 = call-poly <vilib>:"WPI_RobotDriveArcadeDrive.vi"("error in (no error)"=w783, "Y axis value"=w779, "X axis value"=-0.8, "RobotDriveDevRef"=w784) -> ()  [unwired: 5 in, 3 out]
      }
      n258 = while {
        tunnel: w676 -> [w725]
        tunnel: w675 -> [w726]
        tunnel: [w726] -> w674
        tunnel: [w725] -> w673
        i -> [w718]
        stop <- w717 stop-if-true
        n259 = Increment(x=w718) -> (x+1=w720:i32)
        n260 = call <vilib>:"CTRE_PigeonIMU_RefNumRegistryGet.vi"("refnum name"="Pigeon") -> ("error out"=w722:errorcluster, "PigeonIMUDevRef"=w723:T14)  [unwired: 9 in]
        n261 = call <vilib>:"CTRE_PigeonIMU_SetYaw.vi"("error in (no error)"=w722, "Value"=0.0, "PigeonIMUDevRef"=w723) -> ()  [unwired: 7 in, 2 out]
        n262 = Greater?(x=w720, y=10) -> (0:w717:bool)
      }
      n263 = while {
        tunnel: w673 -> [w753]
        tunnel: w674 -> [w752]
        tunnel: [w753] -> w666
        tunnel: [w752] -> w665
        i -> [w758]
        stop <- w757 stop-if-true
        n264 = Increment(x=w758) -> (x+1=w755:i32)
        n265 = Wait (ms)(milliseconds to wait=u32 20) -> ()  [unwired: 1 out]
        n266 = global read "Robot Global Data.vi" "YAW"() -> (w749:dbl)
        n267 = Greater?(x=w755, y=75) -> (0:w757:bool)
        n268 = call-poly <vilib>:"PID.vi"("output range"=cluster{"output high":dbl, "output low":dbl} {"output high"=1.0, "output low"=-1.0}, "PID gains"=T7 {"proportional gain (Kc)"=0.015, "integral time (Ti, min)"=0.0, "derivative time (Td, min)"=0.0}, "process variable"=w749, "setpoint"=-45.0) -> ("output"=w748:dbl)  [unwired: 6 in, 1 out]
        n269 = call-poly <vilib>:"WPI_RobotDriveArcadeDrive.vi"("error in (no error)"=w752, "Y axis value"=w748, "X axis value"=0.0, "RobotDriveDevRef"=w753) -> ()  [unwired: 5 in, 3 out]
      }
      n270 = while {
        tunnel: w666 -> [w681]
        tunnel: w665 -> [w680]
        tunnel: [w681] -> w664
        tunnel: [w680] -> w663
        i -> [w683]
        stop <- w682 stop-if-true
        n271 = Increment(x=w683) -> (x+1=w685:i32)
        n272 = call-poly <vilib>:"WPI_RobotDriveArcadeDrive.vi"("error in (no error)"=w680, "X axis value"=0.3, "RobotDriveDevRef"=w681) -> ()  [unwired: 6 in, 3 out]
        n273 = Greater?(x=w685, y=20) -> (0:w682:bool)
      }
      n274 = while {
        tunnel: w664 -> [w728]
        tunnel: w663 -> [w727]
        tunnel: [w728] -> w668
        tunnel: [w727] -> w667
        i -> [w741]
        stop <- w730 stop-if-true
        w733 = -0.75
        n275 = Increment(x=w741) -> (x+1=w731:i32)
        n276 = call <vilib>:"WPI_MotorControlRefNum Registry Get.vi"("refnum name"="Acquire 2") -> ("error out"=w734:errorcluster, "MotorControlDevRef"=w735:T9)  [unwired: 9 in]
        n277 = call <vilib>:"WPI_MotorControlRefNum Registry Get.vi"("refnum name"="Acquire") -> ("error out"=w737:errorcluster, "MotorControlDevRef"=w738:T9)  [unwired: 9 in]
        n278 = Greater?(x=w731, y=140) -> (0:w729:bool)
        n279 = call <vilib>:"WPI_MotorControlSetOutput.vi"("error in (no error)"=w737, "Output"=w733, "MotorControlDevRef"=w738) -> ()  [unwired: 6 in, 3 out]
        n280 = call <vilib>:"WPI_MotorControlSetOutput.vi"("error in (no error)"=w734, "Output"=w733, "MotorControlDevRef"=w735) -> ()  [unwired: 6 in, 3 out]
        n281 = case shown="True" w729 {
          frame False {
          }
          frame True {
            n282 = call <vilib>:"WPI_SolenoidRefNum Registry Get.vi"("refnum name"="Push") -> ("error out"=w743:errorcluster, "SolenoidDevRef"=w744:T16)  [unwired: 9 in]
            n283 = call-poly <vilib>:"WPI_SolenoidSet.vi"("error in (no error)"=w743, "Value"=WPI_SolenoidValue."Reverse", "SolenoidDevRef"=w744) -> ()  [unwired: 7 in, 2 out]
          }
        }
        n284 = Greater?(x=w731, y=250) -> (0:w730:bool)
      }
      n285 = while {
        tunnel: w668 -> [w688]
        tunnel: w667 -> [w687]
        tunnel: [w688] -> _
        tunnel: [w687] -> _
        i -> [w701]
        stop <- w690 stop-if-true
        w693 = 0.0
        n286 = Increment(x=w701) -> (x+1=w691:i32)
        n287 = call <vilib>:"WPI_MotorControlRefNum Registry Get.vi"("refnum name"="Acquire 2") -> ("error out"=w694:errorcluster, "MotorControlDevRef"=w695:T9)  [unwired: 9 in]
        n288 = call <vilib>:"WPI_MotorControlRefNum Registry Get.vi"("refnum name"="Acquire") -> ("error out"=w697:errorcluster, "MotorControlDevRef"=w698:T9)  [unwired: 9 in]
        n289 = Greater?(x=w691, y=140) -> (0:w689:bool)
        n290 = call <vilib>:"WPI_MotorControlSetOutput.vi"("error in (no error)"=w697, "Output"=w693, "MotorControlDevRef"=w698) -> ()  [unwired: 6 in, 3 out]
        n291 = call <vilib>:"WPI_MotorControlSetOutput.vi"("error in (no error)"=w694, "Output"=w693, "MotorControlDevRef"=w695) -> ()  [unwired: 6 in, 3 out]
        n292 = case shown="True" w689 {
          frame False {
          }
          frame True {
            n293 = call <vilib>:"WPI_SolenoidRefNum Registry Get.vi"("refnum name"="Push") -> ("error out"=w703:errorcluster, "SolenoidDevRef"=w704:T16)  [unwired: 9 in]
            n294 = call-poly <vilib>:"WPI_SolenoidSet.vi"("error in (no error)"=w703, "Value"=WPI_SolenoidValue."Forward", "SolenoidDevRef"=w704) -> ()  [unwired: 7 in, 2 out]
          }
        }
        n295 = Greater?(x=w691, y=250) -> (0:w690:bool)
      }
    }
    frame "Place Switch and Scale Right" {
      n296 = call <vilib>:"WPI_RobotDriveRefNum Registry Get.vi"("refnum name"="TANK") -> ("error out"=w800:errorcluster, "RobotDriveDevRef"=w801:T8)  [unwired: 9 in]
      n297 = while {
        tunnel: [w893] -> w795
        tunnel: w801 -> [w893]
        tunnel: w800 -> [w892]
        tunnel: [w892] -> w794
        i -> [w889]
        stop <- w888 stop-if-true
        n298 = call <vilib>:"CTRE_PigeonIMU_RefNumRegistryGet.vi"("refnum name"="Pigeon") -> ("error out"=w885:errorcluster, "PigeonIMUDevRef"=w886:T14)  [unwired: 9 in]
        n299 = Increment(x=w889) -> (x+1=w890:i32)
        n300 = call <vilib>:"WPI_SolenoidRefNum Registry Get.vi"("refnum name"="Kickers") -> ("error out"=w877:errorcluster, "SolenoidDevRef"=w878:T16)  [unwired: 9 in]
        n301 = call <vilib>:"WPI_SolenoidRefNum Registry Get.vi"("refnum name"="Push") -> ("error out"=w881:errorcluster, "SolenoidDevRef"=w882:T16)  [unwired: 9 in]
        n302 = call <vilib>:"CTRE_PigeonIMU_SetYaw.vi"("error in (no error)"=w885, "Value"=0.0, "PigeonIMUDevRef"=w886) -> ()  [unwired: 7 in, 2 out]
        n303 = Greater?(x=w890, y=15) -> (0:w888:bool)
        n304 = call-poly <vilib>:"WPI_SolenoidSet.vi"("error in (no error)"=w877, "Value"=WPI_SolenoidValue."Reverse", "SolenoidDevRef"=w878) -> ()  [unwired: 7 in, 2 out]
        n305 = call-poly <vilib>:"WPI_SolenoidSet.vi"("error in (no error)"=w881, "Value"=WPI_SolenoidValue."Forward", "SolenoidDevRef"=w882) -> ()  [unwired: 7 in, 2 out]
      }
      n306 = while {
        tunnel: w795 -> [w825]
        tunnel: [w825] -> w793
        tunnel: w794 -> [w824]
        tunnel: [w824] -> w792
        i -> [w827]
        stop <- w826 stop-if-true
        n307 = Increment(x=w827) -> (x+1=w828:i32)
        n308 = global read "Robot Global Data.vi" "YAW"() -> (w833:dbl)
        n309 = call-poly <vilib>:"PID.vi"("output range"=cluster{"output high":dbl, "output low":dbl} {"output high"=1.0, "output low"=-1.0}, "PID gains"=T7 {"proportional gain (Kc)"=0.02, "integral time (Ti, min)"=0.0, "derivative time (Td, min)"=0.0}, "process variable"=w833, "setpoint"=-4.0) -> ("output"=w832:dbl)  [unwired: 6 in, 1 out]
        n310 = Greater?(x=w828, y=40) -> (0:w826:bool)
        n311 = call-poly <vilib>:"WPI_RobotDriveArcadeDrive.vi"("error in (no error)"=w824, "Y axis value"=w832, "X axis value"=0.0, "RobotDriveDevRef"=w825) -> ()  [unwired: 5 in, 3 out]
      }
      n312 = while {
        tunnel: w793 -> [w901]
        tunnel: w792 -> [w900]
        tunnel: [w901] -> w803
        tunnel: [w900] -> w802
        i -> [w903]
        stop <- w906 stop-if-true
        # ".1"
        # ".1"
        # "250"
        # "p=.018\nI=.01\nD=.001"
        n313 = Increment(x=w903) -> (x+1=w902:i32)
        n314 = Wait (ms)(milliseconds to wait=u32 20) -> ()  [unwired: 1 out]
        n315 = Greater?(x=w902, y=90) -> (0:w906:bool)
        n316 = global read "Robot Global Data.vi" "YAW"() -> (w897:dbl)
        n317 = call-poly <vilib>:"PID.vi"("output range"=cluster{"output high":dbl, "output low":dbl} {"output high"=1.0, "output low"=-1.0}, "PID gains"=T7 {"proportional gain (Kc)"=1.0, "integral time (Ti, min)"=0.0, "derivative time (Td, min)"=0.0}, "process variable"=w897, "setpoint"=-4.0) -> ("output"=w895:dbl)  [unwired: 6 in, 1 out]
        n318 = call-poly <vilib>:"WPI_RobotDriveArcadeDrive.vi"("error in (no error)"=w900, "Y axis value"=w895, "X axis value"=-1.0, "RobotDriveDevRef"=w901) -> ()  [unwired: 5 in, 3 out]
      }
      n319 = while {
        tunnel: w803 -> [w870]
        tunnel: w802 -> [w869]
        tunnel: [w870] -> w799
        tunnel: [w869] -> w798
        i -> [w875]
        stop <- w874 stop-if-true
        n320 = Increment(x=w875) -> (x+1=w872:i32)
        n321 = Wait (ms)(milliseconds to wait=u32 20) -> ()  [unwired: 1 out]
        n322 = global read "Robot Global Data.vi" "YAW"() -> (w866:dbl)
        n323 = Greater?(x=w872, y=50) -> (0:w874:bool)
        n324 = call-poly <vilib>:"PID.vi"("output range"=cluster{"output high":dbl, "output low":dbl} {"output high"=1.0, "output low"=-1.0}, "PID gains"=T7 {"proportional gain (Kc)"=0.018, "integral time (Ti, min)"=0.0, "derivative time (Td, min)"=0.0}, "process variable"=w866, "setpoint"=90.0) -> ("output"=w865:dbl)  [unwired: 6 in, 1 out]
        n325 = call-poly <vilib>:"WPI_RobotDriveArcadeDrive.vi"("error in (no error)"=w869, "Y axis value"=w865, "X axis value"=0.0, "RobotDriveDevRef"=w870) -> ()  [unwired: 5 in, 3 out]
      }
      n326 = while {
        tunnel: w799 -> [w858]
        tunnel: w798 -> [w857]
        tunnel: [w858] -> w797
        tunnel: [w857] -> w796
        i -> [w856]
        stop <- w862 stop-if-true
        n327 = Increment(x=w856) -> (x+1=w855:i32)
        n328 = Wait (ms)(milliseconds to wait=u32 20) -> ()  [unwired: 1 out]
        n329 = Greater?(x=w855, y=10) -> (0:w862:bool)
        n330 = call-poly <vilib>:"WPI_RobotDriveArcadeDrive.vi"("error in (no error)"=w857, "X axis value"=-0.8, "RobotDriveDevRef"=w858) -> ()  [unwired: 6 in, 3 out]
      }
      n331 = while {
        tunnel: [w838] -> w791
        tunnel: w797 -> [w838]
        tunnel: [w837] -> w790
        tunnel: w796 -> [w837]
        i -> [w840]
        stop <- w839 stop-if-true
        n332 = call <vilib>:"WPI_SolenoidRefNum Registry Get.vi"("refnum name"="Push") -> ("error out"=w852:errorcluster, "SolenoidDevRef"=w853:T16)  [unwired: 9 in]
        n333 = call <vilib>:"WPI_MotorControlRefNum Registry Get.vi"("refnum name"="Acquire") -> ("error out"=w845:errorcluster, "MotorControlDevRef"=w846:T9)  [unwired: 9 in]
        n334 = call <vilib>:"WPI_MotorControlRefNum Registry Get.vi"("refnum name"="Acquire 2") -> ("error out"=w847:errorcluster, "MotorControlDevRef"=w848:T9)  [unwired: 9 in]
        n335 = Increment(x=w840) -> (x+1=w841:i32)
        n336 = call <vilib>:"WPI_MotorControlSetOutput.vi"("error in (no error)"=w847, "Output"=-0.4, "MotorControlDevRef"=w848) -> ()  [unwired: 6 in, 3 out]
        n337 = call <vilib>:"WPI_MotorControlSetOutput.vi"("error in (no error)"=w845, "Output"=-0.4, "MotorControlDevRef"=w846) -> ()  [unwired: 6 in, 3 out]
        n338 = call-poly <vilib>:"WPI_SolenoidSet.vi"("error in (no error)"=w852, "Value"=WPI_SolenoidValue."Reverse", "SolenoidDevRef"=w853) -> ()  [unwired: 7 in, 2 out]
        n339 = Greater?(x=w841, y=50) -> (0:w839:bool)
        n340 = Wait (ms)(milliseconds to wait=u32 20) -> ()  [unwired: 1 out]
      }
      n341 = while {
        tunnel: [w810] -> _
        tunnel: w791 -> [w810]
        tunnel: [w809] -> _
        tunnel: w790 -> [w809]
        i -> [w813]
        stop <- w812 stop-if-true
        n342 = call <vilib>:"WPI_SolenoidRefNum Registry Get.vi"("refnum name"="Push") -> ("error out"=w806:errorcluster, "SolenoidDevRef"=w807:T16)  [unwired: 9 in]
        n343 = call <vilib>:"WPI_MotorControlRefNum Registry Get.vi"("refnum name"="Acquire") -> ("error out"=w818:errorcluster, "MotorControlDevRef"=w819:T9)  [unwired: 9 in]
        n344 = call <vilib>:"WPI_MotorControlRefNum Registry Get.vi"("refnum name"="Acquire 2") -> ("error out"=w820:errorcluster, "MotorControlDevRef"=w821:T9)  [unwired: 9 in]
        n345 = Increment(x=w813) -> (x+1=w814:i32)
        n346 = call-poly <vilib>:"WPI_SolenoidSet.vi"("error in (no error)"=w806, "Value"=WPI_SolenoidValue."Forward", "SolenoidDevRef"=w807) -> ()  [unwired: 7 in, 2 out]
        n347 = call <vilib>:"WPI_MotorControlSetOutput.vi"("error in (no error)"=w820, "Output"=0.0, "MotorControlDevRef"=w821) -> ()  [unwired: 6 in, 3 out]
        n348 = call <vilib>:"WPI_MotorControlSetOutput.vi"("error in (no error)"=w818, "Output"=0.0, "MotorControlDevRef"=w819) -> ()  [unwired: 6 in, 3 out]
        n349 = Greater?(x=w814, y=100) -> (0:w812:bool)
        n350 = Wait (ms)(milliseconds to wait=u32 20) -> ()  [unwired: 1 out]
      }
    }
    frame "Place 2 Switch Right" {
      # "done"
      n351 = call <vilib>:"WPI_RobotDriveRefNum Registry Get.vi"("refnum name"="TANK") -> ("error out"=w917:errorcluster, "RobotDriveDevRef"=w918:T8)  [unwired: 9 in]
      n352 = while {
        tunnel: [w1010] -> w910
        tunnel: w918 -> [w1010]
        tunnel: w917 -> [w1009]
        tunnel: [w1009] -> w909
        i -> [w1006]
        stop <- w1005 stop-if-true
        n353 = call <vilib>:"CTRE_PigeonIMU_RefNumRegistryGet.vi"("refnum name"="Pigeon") -> ("error out"=w1002:errorcluster, "PigeonIMUDevRef"=w1003:T14)  [unwired: 9 in]
        n354 = Increment(x=w1006) -> (x+1=w1007:i32)
        n355 = call <vilib>:"WPI_SolenoidRefNum Registry Get.vi"("refnum name"="Kickers") -> ("error out"=w994:errorcluster, "SolenoidDevRef"=w995:T16)  [unwired: 9 in]
        n356 = call <vilib>:"WPI_SolenoidRefNum Registry Get.vi"("refnum name"="Push") -> ("error out"=w998:errorcluster, "SolenoidDevRef"=w999:T16)  [unwired: 9 in]
        n357 = call <vilib>:"CTRE_PigeonIMU_SetYaw.vi"("error in (no error)"=w1002, "Value"=0.0, "PigeonIMUDevRef"=w1003) -> ()  [unwired: 7 in, 2 out]
        n358 = Greater?(x=w1007, y=15) -> (0:w1005:bool)
        n359 = call-poly <vilib>:"WPI_SolenoidSet.vi"("error in (no error)"=w994, "Value"=WPI_SolenoidValue."Reverse", "SolenoidDevRef"=w995) -> ()  [unwired: 7 in, 2 out]
        n360 = call-poly <vilib>:"WPI_SolenoidSet.vi"("error in (no error)"=w998, "Value"=WPI_SolenoidValue."Forward", "SolenoidDevRef"=w999) -> ()  [unwired: 7 in, 2 out]
      }
      n361 = while {
        tunnel: w910 -> [w923]
        tunnel: [w923] -> w908
        tunnel: w909 -> [w922]
        tunnel: [w922] -> w907
        i -> [w925]
        stop <- w924 stop-if-true
        n362 = Increment(x=w925) -> (x+1=w926:i32)
        n363 = global read "Robot Global Data.vi" "YAW"() -> (w931:dbl)
        n364 = call-poly <vilib>:"PID.vi"("output range"=cluster{"output high":dbl, "output low":dbl} {"output high"=1.0, "output low"=-1.0}, "PID gains"=T7 {"proportional gain (Kc)"=0.02, "integral time (Ti, min)"=0.0, "derivative time (Td, min)"=0.0}, "process variable"=w931, "setpoint"=0.0) -> ("output"=w930:dbl)  [unwired: 6 in, 1 out]
        n365 = Greater?(x=w926, y=50) -> (0:w924:bool)
        n366 = call-poly <vilib>:"WPI_RobotDriveArcadeDrive.vi"("error in (no error)"=w922, "Y axis value"=w930, "X axis value"=0.0, "RobotDriveDevRef"=w923) -> ()  [unwired: 5 in, 3 out]
      }
      n367 = while {
        tunnel: w908 -> [w1018]
        tunnel: w907 -> [w1017]
        tunnel: [w1018] -> w920
        tunnel: [w1017] -> w919
        i -> [w1020]
        stop <- w1023 stop-if-true
        # ".1"
        # ".1"
        # "250"
        # "p=.018\nI=.01\nD=.001"
        n368 = Increment(x=w1020) -> (x+1=w1019:i32)
        n369 = Wait (ms)(milliseconds to wait=u32 20) -> ()  [unwired: 1 out]
        n370 = Greater?(x=w1019, y=77) -> (0:w1023:bool)
        n371 = global read "Robot Global Data.vi" "YAW"() -> (w1014:dbl)
        n372 = call-poly <vilib>:"PID.vi"("output range"=cluster{"output high":dbl, "output low":dbl} {"output high"=1.0, "output low"=-1.0}, "PID gains"=T7 {"proportional gain (Kc)"=0.1, "integral time (Ti, min)"=0.0, "derivative time (Td, min)"=0.0}, "process variable"=w1014, "setpoint"=0.0) -> ("output"=w1012:dbl)  [unwired: 6 in, 1 out]
        n373 = call-poly <vilib>:"WPI_RobotDriveArcadeDrive.vi"("error in (no error)"=w1017, "Y axis value"=w1012, "X axis value"=-0.8, "RobotDriveDevRef"=w1018) -> ()  [unwired: 5 in, 3 out]
      }
      n374 = while {
        tunnel: w920 -> [w987]
        tunnel: w919 -> [w986]
        tunnel: [w987] -> w916
        tunnel: [w986] -> w915
        i -> [w992]
        stop <- w991 stop-if-true
        n375 = Increment(x=w992) -> (x+1=w989:i32)
        n376 = Wait (ms)(milliseconds to wait=u32 20) -> ()  [unwired: 1 out]
        n377 = global read "Robot Global Data.vi" "YAW"() -> (w983:dbl)
        n378 = Greater?(x=w989, y=60) -> (0:w991:bool)
        n379 = call-poly <vilib>:"PID.vi"("output range"=cluster{"output high":dbl, "output low":dbl} {"output high"=0.8, "output low"=-0.8}, "PID gains"=T7 {"proportional gain (Kc)"=0.015, "integral time (Ti, min)"=0.0, "derivative time (Td, min)"=0.0}, "process variable"=w983, "setpoint"=-90.0) -> ("output"=w982:dbl)  [unwired: 6 in, 1 out]
        n380 = call-poly <vilib>:"WPI_RobotDriveArcadeDrive.vi"("error in (no error)"=w986, "Y axis value"=w982, "X axis value"=0.0, "RobotDriveDevRef"=w987) -> ()  [unwired: 5 in, 3 out]
      }
      n381 = while {
        tunnel: w916 -> [w975]
        tunnel: w915 -> [w974]
        tunnel: [w975] -> w914
        tunnel: [w974] -> w913
        i -> [w973]
        stop <- w979 stop-if-true
        n382 = Increment(x=w973) -> (x+1=w972:i32)
        n383 = Wait (ms)(milliseconds to wait=u32 20) -> ()  [unwired: 1 out]
        n384 = Greater?(x=w972, y=22) -> (0:w979:bool)
        n385 = call-poly <vilib>:"WPI_RobotDriveArcadeDrive.vi"("error in (no error)"=w974, "X axis value"=-0.8, "RobotDriveDevRef"=w975) -> ()  [unwired: 6 in, 3 out]
      }
      n386 = while {
        tunnel: [w955] -> w912
        tunnel: w914 -> [w955]
        tunnel: [w954] -> w911
        tunnel: w913 -> [w954]
        i -> [w957]
        stop <- w956 stop-if-true
        n387 = call <vilib>:"WPI_SolenoidRefNum Registry Get.vi"("refnum name"="Push") -> ("error out"=w969:errorcluster, "SolenoidDevRef"=w970:T16)  [unwired: 9 in]
        n388 = call <vilib>:"WPI_MotorControlRefNum Registry Get.vi"("refnum name"="Acquire") -> ("error out"=w962:errorcluster, "MotorControlDevRef"=w963:T9)  [unwired: 9 in]
        n389 = call <vilib>:"WPI_MotorControlRefNum Registry Get.vi"("refnum name"="Acquire 2") -> ("error out"=w964:errorcluster, "MotorControlDevRef"=w965:T9)  [unwired: 9 in]
        n390 = Increment(x=w957) -> (x+1=w958:i32)
        n391 = call <vilib>:"WPI_MotorControlSetOutput.vi"("error in (no error)"=w964, "Output"=-0.3, "MotorControlDevRef"=w965) -> ()  [unwired: 6 in, 3 out]
        n392 = call <vilib>:"WPI_MotorControlSetOutput.vi"("error in (no error)"=w962, "Output"=-0.3, "MotorControlDevRef"=w963) -> ()  [unwired: 6 in, 3 out]
        n393 = call-poly <vilib>:"WPI_SolenoidSet.vi"("error in (no error)"=w969, "Value"=WPI_SolenoidValue."Reverse", "SolenoidDevRef"=w970) -> ()  [unwired: 7 in, 2 out]
        n394 = Greater?(x=w958, y=50) -> (0:w956:bool)
        n395 = Wait (ms)(milliseconds to wait=u32 20) -> ()  [unwired: 1 out]
      }
      n396 = while {
        tunnel: [w939] -> _
        tunnel: w912 -> [w939]
        tunnel: [w938] -> _
        tunnel: w911 -> [w938]
        i -> [w942]
        stop <- w941 stop-if-true
        n397 = call <vilib>:"WPI_SolenoidRefNum Registry Get.vi"("refnum name"="Push") -> ("error out"=w935:errorcluster, "SolenoidDevRef"=w936:T16)  [unwired: 9 in]
        n398 = call <vilib>:"WPI_MotorControlRefNum Registry Get.vi"("refnum name"="Acquire") -> ("error out"=w947:errorcluster, "MotorControlDevRef"=w948:T9)  [unwired: 9 in]
        n399 = call <vilib>:"WPI_MotorControlRefNum Registry Get.vi"("refnum name"="Acquire 2") -> ("error out"=w949:errorcluster, "MotorControlDevRef"=w950:T9)  [unwired: 9 in]
        n400 = Increment(x=w942) -> (x+1=w943:i32)
        n401 = call-poly <vilib>:"WPI_SolenoidSet.vi"("error in (no error)"=w935, "Value"=WPI_SolenoidValue."Forward", "SolenoidDevRef"=w936) -> ()  [unwired: 7 in, 2 out]
        n402 = call <vilib>:"WPI_MotorControlSetOutput.vi"("error in (no error)"=w949, "Output"=0.0, "MotorControlDevRef"=w950) -> ()  [unwired: 6 in, 3 out]
        n403 = call <vilib>:"WPI_MotorControlSetOutput.vi"("error in (no error)"=w947, "Output"=0.0, "MotorControlDevRef"=w948) -> ()  [unwired: 6 in, 3 out]
        n404 = Greater?(x=w943, y=100) -> (0:w941:bool)
        n405 = Wait (ms)(milliseconds to wait=u32 20) -> ()  [unwired: 1 out]
      }
    }
    frame "Place 2 Switch Left" {
      # "done"
      n406 = call <vilib>:"WPI_RobotDriveRefNum Registry Get.vi"("refnum name"="TANK") -> ("error out"=w1034:errorcluster, "RobotDriveDevRef"=w1035:T8)  [unwired: 9 in]
      n407 = while {
        tunnel: [w1127] -> w1027
        tunnel: w1035 -> [w1127]
        tunnel: w1034 -> [w1126]
        tunnel: [w1126] -> w1026
        i -> [w1123]
        stop <- w1122 stop-if-true
        n408 = call <vilib>:"CTRE_PigeonIMU_RefNumRegistryGet.vi"("refnum name"="Pigeon") -> ("error out"=w1119:errorcluster, "PigeonIMUDevRef"=w1120:T14)  [unwired: 9 in]
        n409 = Increment(x=w1123) -> (x+1=w1124:i32)
        n410 = call <vilib>:"WPI_SolenoidRefNum Registry Get.vi"("refnum name"="Kickers") -> ("error out"=w1111:errorcluster, "SolenoidDevRef"=w1112:T16)  [unwired: 9 in]
        n411 = call <vilib>:"WPI_SolenoidRefNum Registry Get.vi"("refnum name"="Push") -> ("error out"=w1115:errorcluster, "SolenoidDevRef"=w1116:T16)  [unwired: 9 in]
        n412 = call <vilib>:"CTRE_PigeonIMU_SetYaw.vi"("error in (no error)"=w1119, "Value"=0.0, "PigeonIMUDevRef"=w1120) -> ()  [unwired: 7 in, 2 out]
        n413 = Greater?(x=w1124, y=15) -> (0:w1122:bool)
        n414 = call-poly <vilib>:"WPI_SolenoidSet.vi"("error in (no error)"=w1111, "Value"=WPI_SolenoidValue."Reverse", "SolenoidDevRef"=w1112) -> ()  [unwired: 7 in, 2 out]
        n415 = call-poly <vilib>:"WPI_SolenoidSet.vi"("error in (no error)"=w1115, "Value"=WPI_SolenoidValue."Forward", "SolenoidDevRef"=w1116) -> ()  [unwired: 7 in, 2 out]
      }
      n416 = while {
        tunnel: w1027 -> [w1040]
        tunnel: [w1040] -> w1025
        tunnel: w1026 -> [w1039]
        tunnel: [w1039] -> w1024
        i -> [w1042]
        stop <- w1041 stop-if-true
        n417 = Increment(x=w1042) -> (x+1=w1043:i32)
        n418 = global read "Robot Global Data.vi" "YAW"() -> (w1048:dbl)
        n419 = call-poly <vilib>:"PID.vi"("output range"=cluster{"output high":dbl, "output low":dbl} {"output high"=1.0, "output low"=-1.0}, "PID gains"=T7 {"proportional gain (Kc)"=0.02, "integral time (Ti, min)"=0.0, "derivative time (Td, min)"=0.0}, "process variable"=w1048, "setpoint"=0.0) -> ("output"=w1047:dbl)  [unwired: 6 in, 1 out]
        n420 = Greater?(x=w1043, y=50) -> (0:w1041:bool)
        n421 = call-poly <vilib>:"WPI_RobotDriveArcadeDrive.vi"("error in (no error)"=w1039, "Y axis value"=w1047, "X axis value"=0.0, "RobotDriveDevRef"=w1040) -> ()  [unwired: 5 in, 3 out]
      }
      n422 = while {
        tunnel: w1025 -> [w1135]
        tunnel: w1024 -> [w1134]
        tunnel: [w1135] -> w1037
        tunnel: [w1134] -> w1036
        i -> [w1137]
        stop <- w1140 stop-if-true
        # ".1"
        # ".1"
        # "250"
        # "p=.018\nI=.01\nD=.001"
        n423 = Increment(x=w1137) -> (x+1=w1136:i32)
        n424 = Wait (ms)(milliseconds to wait=u32 20) -> ()  [unwired: 1 out]
        n425 = Greater?(x=w1136, y=77) -> (0:w1140:bool)
        n426 = global read "Robot Global Data.vi" "YAW"() -> (w1131:dbl)
        n427 = call-poly <vilib>:"PID.vi"("output range"=cluster{"output high":dbl, "output low":dbl} {"output high"=1.0, "output low"=-1.0}, "PID gains"=T7 {"proportional gain (Kc)"=0.1, "integral time (Ti, min)"=0.0, "derivative time (Td, min)"=0.0}, "process variable"=w1131, "setpoint"=0.0) -> ("output"=w1129:dbl)  [unwired: 6 in, 1 out]
        n428 = call-poly <vilib>:"WPI_RobotDriveArcadeDrive.vi"("error in (no error)"=w1134, "Y axis value"=w1129, "X axis value"=-0.8, "RobotDriveDevRef"=w1135) -> ()  [unwired: 5 in, 3 out]
      }
      n429 = while {
        tunnel: w1037 -> [w1104]
        tunnel: w1036 -> [w1103]
        tunnel: [w1104] -> w1033
        tunnel: [w1103] -> w1032
        i -> [w1109]
        stop <- w1108 stop-if-true
        n430 = Increment(x=w1109) -> (x+1=w1106:i32)
        n431 = Wait (ms)(milliseconds to wait=u32 20) -> ()  [unwired: 1 out]
        n432 = global read "Robot Global Data.vi" "YAW"() -> (w1100:dbl)
        n433 = Greater?(x=w1106, y=60) -> (0:w1108:bool)
        n434 = call-poly <vilib>:"PID.vi"("output range"=cluster{"output high":dbl, "output low":dbl} {"output high"=0.8, "output low"=-0.8}, "PID gains"=T7 {"proportional gain (Kc)"=0.015, "integral time (Ti, min)"=0.0, "derivative time (Td, min)"=0.0}, "process variable"=w1100, "setpoint"=90.0) -> ("output"=w1099:dbl)  [unwired: 6 in, 1 out]
        n435 = call-poly <vilib>:"WPI_RobotDriveArcadeDrive.vi"("error in (no error)"=w1103, "Y axis value"=w1099, "X axis value"=0.0, "RobotDriveDevRef"=w1104) -> ()  [unwired: 5 in, 3 out]
      }
      n436 = while {
        tunnel: w1033 -> [w1092]
        tunnel: w1032 -> [w1091]
        tunnel: [w1092] -> w1031
        tunnel: [w1091] -> w1030
        i -> [w1090]
        stop <- w1096 stop-if-true
        n437 = Increment(x=w1090) -> (x+1=w1089:i32)
        n438 = Wait (ms)(milliseconds to wait=u32 20) -> ()  [unwired: 1 out]
        n439 = Greater?(x=w1089, y=22) -> (0:w1096:bool)
        n440 = call-poly <vilib>:"WPI_RobotDriveArcadeDrive.vi"("error in (no error)"=w1091, "X axis value"=-0.8, "RobotDriveDevRef"=w1092) -> ()  [unwired: 6 in, 3 out]
      }
      n441 = while {
        tunnel: [w1072] -> w1029
        tunnel: w1031 -> [w1072]
        tunnel: [w1071] -> w1028
        tunnel: w1030 -> [w1071]
        i -> [w1074]
        stop <- w1073 stop-if-true
        n442 = call <vilib>:"WPI_SolenoidRefNum Registry Get.vi"("refnum name"="Push") -> ("error out"=w1086:errorcluster, "SolenoidDevRef"=w1087:T16)  [unwired: 9 in]
        n443 = call <vilib>:"WPI_MotorControlRefNum Registry Get.vi"("refnum name"="Acquire") -> ("error out"=w1079:errorcluster, "MotorControlDevRef"=w1080:T9)  [unwired: 9 in]
        n444 = call <vilib>:"WPI_MotorControlRefNum Registry Get.vi"("refnum name"="Acquire 2") -> ("error out"=w1081:errorcluster, "MotorControlDevRef"=w1082:T9)  [unwired: 9 in]
        n445 = Increment(x=w1074) -> (x+1=w1075:i32)
        n446 = call <vilib>:"WPI_MotorControlSetOutput.vi"("error in (no error)"=w1081, "Output"=-0.3, "MotorControlDevRef"=w1082) -> ()  [unwired: 6 in, 3 out]
        n447 = call <vilib>:"WPI_MotorControlSetOutput.vi"("error in (no error)"=w1079, "Output"=-0.3, "MotorControlDevRef"=w1080) -> ()  [unwired: 6 in, 3 out]
        n448 = call-poly <vilib>:"WPI_SolenoidSet.vi"("error in (no error)"=w1086, "Value"=WPI_SolenoidValue."Reverse", "SolenoidDevRef"=w1087) -> ()  [unwired: 7 in, 2 out]
        n449 = Greater?(x=w1075, y=50) -> (0:w1073:bool)
        n450 = Wait (ms)(milliseconds to wait=u32 20) -> ()  [unwired: 1 out]
      }
      n451 = while {
        tunnel: [w1056] -> _
        tunnel: w1029 -> [w1056]
        tunnel: [w1055] -> _
        tunnel: w1028 -> [w1055]
        i -> [w1059]
        stop <- w1058 stop-if-true
        n452 = call <vilib>:"WPI_SolenoidRefNum Registry Get.vi"("refnum name"="Push") -> ("error out"=w1052:errorcluster, "SolenoidDevRef"=w1053:T16)  [unwired: 9 in]
        n453 = call <vilib>:"WPI_MotorControlRefNum Registry Get.vi"("refnum name"="Acquire") -> ("error out"=w1064:errorcluster, "MotorControlDevRef"=w1065:T9)  [unwired: 9 in]
        n454 = call <vilib>:"WPI_MotorControlRefNum Registry Get.vi"("refnum name"="Acquire 2") -> ("error out"=w1066:errorcluster, "MotorControlDevRef"=w1067:T9)  [unwired: 9 in]
        n455 = Increment(x=w1059) -> (x+1=w1060:i32)
        n456 = call-poly <vilib>:"WPI_SolenoidSet.vi"("error in (no error)"=w1052, "Value"=WPI_SolenoidValue."Forward", "SolenoidDevRef"=w1053) -> ()  [unwired: 7 in, 2 out]
        n457 = call <vilib>:"WPI_MotorControlSetOutput.vi"("error in (no error)"=w1066, "Output"=0.0, "MotorControlDevRef"=w1067) -> ()  [unwired: 6 in, 3 out]
        n458 = call <vilib>:"WPI_MotorControlSetOutput.vi"("error in (no error)"=w1064, "Output"=0.0, "MotorControlDevRef"=w1065) -> ()  [unwired: 6 in, 3 out]
        n459 = Greater?(x=w1060, y=100) -> (0:w1058:bool)
        n460 = Wait (ms)(milliseconds to wait=u32 20) -> ()  [unwired: 1 out]
      }
    }
    frame "Center Place 1 Switch Right" {
    }
    frame "Center Place 2 Switch Left" {
    }
    frame "Center Place 1 Switch Left" {
    }
    frame "Do Nothing" {
      # "WHOO NOTHING."
    }
    frame "Center Place 2 Switch Right" {
    }
    frame "Place Scale Left" {
      # "done"
      n461 = call <vilib>:"WPI_RobotDriveRefNum Registry Get.vi"("refnum name"="TANK") -> ("error out"=w1155:errorcluster, "RobotDriveDevRef"=w1156:T8)  [unwired: 9 in]
      n462 = while {
        tunnel: [w1254] -> w1150
        tunnel: w1156 -> [w1254]
        tunnel: w1155 -> [w1253]
        tunnel: [w1253] -> w1148
        i -> [w1250]
        stop <- w1249 stop-if-true
        n463 = call <vilib>:"CTRE_PigeonIMU_RefNumRegistryGet.vi"("refnum name"="Pigeon") -> ("error out"=w1246:errorcluster, "PigeonIMUDevRef"=w1247:T14)  [unwired: 9 in]
        n464 = Increment(x=w1250) -> (x+1=w1251:i32)
        n465 = call <vilib>:"WPI_SolenoidRefNum Registry Get.vi"("refnum name"="Kickers") -> ("error out"=w1238:errorcluster, "SolenoidDevRef"=w1239:T16)  [unwired: 9 in]
        n466 = call <vilib>:"WPI_SolenoidRefNum Registry Get.vi"("refnum name"="Push") -> ("error out"=w1242:errorcluster, "SolenoidDevRef"=w1243:T16)  [unwired: 9 in]
        n467 = call <vilib>:"CTRE_PigeonIMU_SetYaw.vi"("error in (no error)"=w1246, "Value"=0.0, "PigeonIMUDevRef"=w1247) -> ()  [unwired: 7 in, 2 out]
        n468 = Greater?(x=w1251, y=15) -> (0:w1249:bool)
        n469 = call-poly <vilib>:"WPI_SolenoidSet.vi"("error in (no error)"=w1238, "Value"=WPI_SolenoidValue."Reverse", "SolenoidDevRef"=w1239) -> ()  [unwired: 7 in, 2 out]
        n470 = call-poly <vilib>:"WPI_SolenoidSet.vi"("error in (no error)"=w1242, "Value"=WPI_SolenoidValue."Forward", "SolenoidDevRef"=w1243) -> ()  [unwired: 7 in, 2 out]
      }
      n471 = while {
        tunnel: w1150 -> [w1188]
        tunnel: [w1188] -> w1149
        tunnel: w1148 -> [w1187]
        tunnel: [w1187] -> w1147
        i -> [w1190]
        stop <- w1189 stop-if-true
        n472 = Increment(x=w1190) -> (x+1=w1191:i32)
        n473 = global read "Robot Global Data.vi" "YAW"() -> (w1185:dbl)
        n474 = call-poly <vilib>:"PID.vi"("output range"=cluster{"output high":dbl, "output low":dbl} {"output high"=1.0, "output low"=-1.0}, "PID gains"=T7 {"proportional gain (Kc)"=0.02, "integral time (Ti, min)"=0.0, "derivative time (Td, min)"=0.0}, "process variable"=w1185, "setpoint"=0.0) -> ("output"=w1186:dbl)  [unwired: 6 in, 1 out]
        n475 = Greater?(x=w1191, y=40) -> (0:w1189:bool)
        n476 = call-poly <vilib>:"WPI_RobotDriveArcadeDrive.vi"("error in (no error)"=w1187, "Y axis value"=w1186, "RobotDriveDevRef"=w1188) -> ()  [unwired: 6 in, 3 out]
      }
      n477 = while {
        tunnel: w1149 -> [w1262]
        tunnel: w1147 -> [w1261]
        tunnel: [w1262] -> w1154
        tunnel: [w1261] -> w1153
        i -> [w1264]
        stop <- w1267 stop-if-true
        # ".1"
        # ".1"
        # "250"
        # "p=.018\nI=.01\nD=.001"
        n478 = Increment(x=w1264) -> (x+1=w1263:i32)
        n479 = Wait (ms)(milliseconds to wait=u32 20) -> ()  [unwired: 1 out]
        n480 = Greater?(x=w1263, y=127) -> (0:w1267:bool)
        n481 = global read "Robot Global Data.vi" "YAW"() -> (w1255:dbl)
        n482 = call-poly <vilib>:"PID.vi"("output range"=cluster{"output high":dbl, "output low":dbl} {"output high"=1.0, "output low"=-1.0}, "PID gains"=T7 {"proportional gain (Kc)"=0.1, "integral time (Ti, min)"=0.0, "derivative time (Td, min)"=0.0}, "process variable"=w1255, "setpoint"=0.0) -> ("output"=w1257:dbl)  [unwired: 6 in, 1 out]
        n483 = call-poly <vilib>:"WPI_RobotDriveArcadeDrive.vi"("error in (no error)"=w1261, "Y axis value"=w1257, "X axis value"=-0.8, "RobotDriveDevRef"=w1262) -> ()  [unwired: 5 in, 3 out]
      }
      n484 = while {
        tunnel: w1154 -> [w1203]
        tunnel: w1153 -> [w1204]
        tunnel: [w1204] -> w1152
        tunnel: [w1203] -> w1151
        i -> [w1196]
        stop <- w1195 stop-if-true
        n485 = Increment(x=w1196) -> (x+1=w1198:i32)
        n486 = call <vilib>:"CTRE_PigeonIMU_RefNumRegistryGet.vi"("refnum name"="Pigeon") -> ("error out"=w1200:errorcluster, "PigeonIMUDevRef"=w1201:T14)  [unwired: 9 in]
        n487 = call <vilib>:"CTRE_PigeonIMU_SetYaw.vi"("error in (no error)"=w1200, "Value"=0.0, "PigeonIMUDevRef"=w1201) -> ()  [unwired: 7 in, 2 out]
        n488 = Greater?(x=w1198, y=10) -> (0:w1195:bool)
      }
      n489 = while {
        tunnel: w1151 -> [w1224]
        tunnel: w1152 -> [w1231]
        tunnel: [w1224] -> w1144
        tunnel: [w1231] -> w1143
        i -> [w1236]
        stop <- w1235 stop-if-true
        n490 = Increment(x=w1236) -> (x+1=w1233:i32)
        n491 = Wait (ms)(milliseconds to wait=u32 20) -> ()  [unwired: 1 out]
        n492 = global read "Robot Global Data.vi" "YAW"() -> (w1228:dbl)
        n493 = Greater?(x=w1233, y=75) -> (0:w1235:bool)
        n494 = call-poly <vilib>:"PID.vi"("output range"=cluster{"output high":dbl, "output low":dbl} {"output high"=1.0, "output low"=-1.0}, "PID gains"=T7 {"proportional gain (Kc)"=0.015, "integral time (Ti, min)"=0.0, "derivative time (Td, min)"=0.0}, "process variable"=w1228, "setpoint"=45.0) -> ("output"=w1227:dbl)  [unwired: 6 in, 1 out]
        n495 = call-poly <vilib>:"WPI_RobotDriveArcadeDrive.vi"("error in (no error)"=w1231, "Y axis value"=w1227, "X axis value"=0.0, "RobotDriveDevRef"=w1224) -> ()  [unwired: 5 in, 3 out]
      }
      n496 = while {
        tunnel: w1144 -> [w1159]
        tunnel: w1143 -> [w1158]
        tunnel: [w1159] -> w1142
        tunnel: [w1158] -> w1141
        i -> [w1161]
        stop <- w1160 stop-if-true
        n497 = Increment(x=w1161) -> (x+1=w1163:i32)
        n498 = call-poly <vilib>:"WPI_RobotDriveArcadeDrive.vi"("error in (no error)"=w1158, "X axis value"=0.3, "RobotDriveDevRef"=w1159) -> ()  [unwired: 6 in, 3 out]
        n499 = Greater?(x=w1163, y=20) -> (0:w1160:bool)
      }
      n500 = while {
        tunnel: w1142 -> [w1206]
        tunnel: w1141 -> [w1205]
        tunnel: [w1206] -> w1146
        tunnel: [w1205] -> w1145
        i -> [w1219]
        stop <- w1208 stop-if-true
        w1211 = -0.75
        n501 = Increment(x=w1219) -> (x+1=w1209:i32)
        n502 = call <vilib>:"WPI_MotorControlRefNum Registry Get.vi"("refnum name"="Acquire 2") -> ("error out"=w1212:errorcluster, "MotorControlDevRef"=w1213:T9)  [unwired: 9 in]
        n503 = call <vilib>:"WPI_MotorControlRefNum Registry Get.vi"("refnum name"="Acquire") -> ("error out"=w1215:errorcluster, "MotorControlDevRef"=w1216:T9)  [unwired: 9 in]
        n504 = Greater?(x=w1209, y=140) -> (0:w1207:bool)
        n505 = call <vilib>:"WPI_MotorControlSetOutput.vi"("error in (no error)"=w1215, "Output"=w1211, "MotorControlDevRef"=w1216) -> ()  [unwired: 6 in, 3 out]
        n506 = call <vilib>:"WPI_MotorControlSetOutput.vi"("error in (no error)"=w1212, "Output"=w1211, "MotorControlDevRef"=w1213) -> ()  [unwired: 6 in, 3 out]
        n507 = case shown="True" w1207 {
          frame False {
          }
          frame True {
            n508 = call <vilib>:"WPI_SolenoidRefNum Registry Get.vi"("refnum name"="Push") -> ("error out"=w1221:errorcluster, "SolenoidDevRef"=w1222:T16)  [unwired: 9 in]
            n509 = call-poly <vilib>:"WPI_SolenoidSet.vi"("error in (no error)"=w1221, "Value"=WPI_SolenoidValue."Reverse", "SolenoidDevRef"=w1222) -> ()  [unwired: 7 in, 2 out]
          }
        }
        n510 = Greater?(x=w1209, y=250) -> (0:w1208:bool)
      }
      n511 = while {
        tunnel: w1146 -> [w1166]
        tunnel: w1145 -> [w1165]
        tunnel: [w1166] -> _
        tunnel: [w1165] -> _
        i -> [w1179]
        stop <- w1168 stop-if-true
        w1171 = 0.0
        n512 = Increment(x=w1179) -> (x+1=w1169:i32)
        n513 = call <vilib>:"WPI_MotorControlRefNum Registry Get.vi"("refnum name"="Acquire 2") -> ("error out"=w1172:errorcluster, "MotorControlDevRef"=w1173:T9)  [unwired: 9 in]
        n514 = call <vilib>:"WPI_MotorControlRefNum Registry Get.vi"("refnum name"="Acquire") -> ("error out"=w1175:errorcluster, "MotorControlDevRef"=w1176:T9)  [unwired: 9 in]
        n515 = Greater?(x=w1169, y=140) -> (0:w1167:bool)
        n516 = call <vilib>:"WPI_MotorControlSetOutput.vi"("error in (no error)"=w1175, "Output"=w1171, "MotorControlDevRef"=w1176) -> ()  [unwired: 6 in, 3 out]
        n517 = call <vilib>:"WPI_MotorControlSetOutput.vi"("error in (no error)"=w1172, "Output"=w1171, "MotorControlDevRef"=w1173) -> ()  [unwired: 6 in, 3 out]
        n518 = case shown="True" w1167 {
          frame False {
          }
          frame True {
            n519 = call <vilib>:"WPI_SolenoidRefNum Registry Get.vi"("refnum name"="Push") -> ("error out"=w1181:errorcluster, "SolenoidDevRef"=w1182:T16)  [unwired: 9 in]
            n520 = call-poly <vilib>:"WPI_SolenoidSet.vi"("error in (no error)"=w1181, "Value"=WPI_SolenoidValue."Forward", "SolenoidDevRef"=w1182) -> ()  [unwired: 7 in, 2 out]
          }
        }
        n521 = Greater?(x=w1169, y=250) -> (0:w1168:bool)
      }
    }
    frame "Place Switch and Scale Left" {
    }
    frame "Drive forward" {
      # "done"
      n522 = call <vilib>:"WPI_RobotDriveRefNum Registry Get.vi"("refnum name"="TANK") -> ("error out"=w1274:errorcluster, "RobotDriveDevRef"=w1275:T8)  [unwired: 9 in]
      n523 = while {
        tunnel: [w1314] -> w1271
        tunnel: w1275 -> [w1314]
        tunnel: w1274 -> [w1313]
        tunnel: [w1313] -> w1269
        i -> [w1310]
        stop <- w1309 stop-if-true
        n524 = call <vilib>:"CTRE_PigeonIMU_RefNumRegistryGet.vi"("refnum name"="Pigeon") -> ("error out"=w1306:errorcluster, "PigeonIMUDevRef"=w1307:T14)  [unwired: 9 in]
        n525 = Increment(x=w1310) -> (x+1=w1311:i32)
        n526 = call <vilib>:"WPI_SolenoidRefNum Registry Get.vi"("refnum name"="Kickers") -> ("error out"=w1298:errorcluster, "SolenoidDevRef"=w1299:T16)  [unwired: 9 in]
        n527 = call <vilib>:"WPI_SolenoidRefNum Registry Get.vi"("refnum name"="Push") -> ("error out"=w1302:errorcluster, "SolenoidDevRef"=w1303:T16)  [unwired: 9 in]
        n528 = call <vilib>:"CTRE_PigeonIMU_SetYaw.vi"("error in (no error)"=w1306, "Value"=0.0, "PigeonIMUDevRef"=w1307) -> ()  [unwired: 7 in, 2 out]
        n529 = Greater?(x=w1311, y=15) -> (0:w1309:bool)
        n530 = call-poly <vilib>:"WPI_SolenoidSet.vi"("error in (no error)"=w1298, "Value"=WPI_SolenoidValue."Reverse", "SolenoidDevRef"=w1299) -> ()  [unwired: 7 in, 2 out]
        n531 = call-poly <vilib>:"WPI_SolenoidSet.vi"("error in (no error)"=w1302, "Value"=WPI_SolenoidValue."Forward", "SolenoidDevRef"=w1303) -> ()  [unwired: 7 in, 2 out]
      }
      n532 = while {
        tunnel: [w1290] -> w1270
        tunnel: w1271 -> [w1290]
        tunnel: w1269 -> [w1289]
        tunnel: [w1289] -> w1268
        i -> [w1286]
        stop <- w1285 stop-if-true
        n533 = global read "Robot Global Data.vi" "YAW"() -> (w1294:dbl)
        n534 = Increment(x=w1286) -> (x+1=w1287:i32)
        n535 = call-poly <vilib>:"PID.vi"("output range"=cluster{"output high":dbl, "output low":dbl} {"output high"=1.0, "output low"=-1.0}, "PID gains"=T7 {"proportional gain (Kc)"=0.02, "integral time (Ti, min)"=0.0, "derivative time (Td, min)"=0.0}, "process variable"=w1294, "setpoint"=0.0) -> ("output"=w1292:dbl)  [unwired: 6 in, 1 out]
        n536 = Greater?(x=w1287, y=50) -> (0:w1285:bool)
        n537 = call-poly <vilib>:"WPI_RobotDriveArcadeDrive.vi"("error in (no error)"=w1289, "Y axis value"=w1292, "X axis value"=0.0, "RobotDriveDevRef"=w1290) -> ()  [unwired: 5 in, 3 out]
      }
      n538 = while {
        tunnel: w1270 -> [w1322]
        tunnel: w1268 -> [w1321]
        tunnel: [w1322] -> w1273
        tunnel: [w1321] -> w1272
        i -> [w1324]
        stop <- w1327 stop-if-true
        # ".1"
        # ".1"
        # "250"
        # "p=.018\nI=.01\nD=.001"
        n539 = Increment(x=w1324) -> (x+1=w1323:i32)
        n540 = Wait (ms)(milliseconds to wait=u32 20) -> ()  [unwired: 1 out]
        n541 = Greater?(x=w1323, y=35) -> (0:w1327:bool)
        n542 = global read "Robot Global Data.vi" "YAW"() -> (w1318:dbl)
        n543 = call-poly <vilib>:"PID.vi"("output range"=cluster{"output high":dbl, "output low":dbl} {"output high"=1.0, "output low"=-1.0}, "PID gains"=T7 {"proportional gain (Kc)"=0.1, "integral time (Ti, min)"=0.0, "derivative time (Td, min)"=0.0}, "process variable"=w1318, "setpoint"=0.0) -> ("output"=w1316:dbl)  [unwired: 6 in, 1 out]
        n544 = call-poly <vilib>:"WPI_RobotDriveArcadeDrive.vi"("error in (no error)"=w1321, "Y axis value"=w1316, "X axis value"=-0.8, "RobotDriveDevRef"=w1322) -> ()  [unwired: 5 in, 3 out]
      }
      n545 = while {
        tunnel: w1273 -> [w1280]
        tunnel: w1272 -> [w1279]
        tunnel: [w1280] -> _
        tunnel: [w1279] -> _
        i -> [w1282]
        stop <- w1284 stop-if-true
        n546 = Increment(x=w1282) -> (x+1=w1281:i32)
        n547 = Greater?(x=w1281, y=97) -> (0:w1284:bool)
        n548 = call-poly <vilib>:"WPI_RobotDriveArcadeDrive.vi"("error in (no error)"=w1279, "Y axis value"=0.0, "X axis value"=0.0, "RobotDriveDevRef"=w1280) -> ()  [unwired: 5 in, 3 out]
      }
    }
  }
  n549 = Format Into String(w11) -> (resulting string=→"Robots Decision 2":string)  [unwired: 3 in, 1 out]
  n550 = while {
    stop <- FALSE stop-if-true
    n551 = call <vilib>:"WPI_DriverStationReport Robot Code State.vi"("Autonomous"=TRUE) -> ()  [unwired: 10 in, 1 out]
    n552 = Wait (ms)(milliseconds to wait=u32 20) -> ()  [unwired: 1 out]
  }
  n553 = call <vilib>:"WPI_DriverStationGet Alliance Info.vi"() -> ()  [unwired: 12 out]
  n554 = call <vilib>:"WPI_JoystickRefNum Registry Get.vi"("refnum name"="Joystick 0") -> ("JoystickDevRef"=w49:T2)  [unwired: 1 in, 9 out]
  n555 = call <vilib>:"WPI_JoystickGetValues.vi"("JoystickDevRef"=w49) -> ("Axes"=w46:dbl[])  [unwired: 6 in, 4 out]
  n556 = call-poly <vilib>:"NT Read Value.vi"("Name"="Auto Selector") -> ()  [unwired: 9 in, 2 out]
  n557 = call-poly <vilib>:"NT Write Value.vi"("Numeric Array"=w46, "Name"="Joystick 0/Axes") -> ()  [unwired: 9 in, 1 out]
  n558 = Index Array(array=w46, index=2) -> ()  [unwired: 1 out]
